vi "MC_7_12f_JW.vi"() -> ()   [LabVIEW 2011]
uses:
  <vilib>/Utility/file.llb/Read From Spreadsheet File (string).vi
  <vilib>/Utility/inputDevices.llb/keyboardAcquire.vi
  <vilib>/Utility/file.llb/Write To Spreadsheet File (DBL).vi
  <vilib>/Utility/file.llb/Write To Spreadsheet File (string).vi
  <vilib>/regexp/Match Regular Expression.xnode
panel:
  out "Rec: Temp":dbl
  out "Comments":string
  out "Folder Index":dbl caption="Length"
  out "Current \nRecord":string[](array[string])
  out "Transformer \nHeaders":string[](array[string])
  out "Current Device ID":string
  out "Column":string
  out "Row":string
  out "Rec: Concentration":dbl
  out "Rec: Solvent":string
  out "Rec: Method":string
  in  "?":T1(tab)
  out "Rec: Material":string
  in  "Treatment Concentration (mM):":dbl=30.0
  in  "Surface Treatment:":string
  in  "# Drops*:":dbl=inf
  in  "Solution Temp (C):":dbl=55.0
  in  "Relative Humidity (%):":dbl=nan
  in  "Room Temp (F):":dbl=nan
  in  "Time (s):":dbl=80.0
  out "Accel (RPM/s):":dbl
  in  "RPM:":dbl=1000.0
  in  "Wait Time (s):":dbl=10.0
  in  "Sample #:":dbl=1.0
  in  "Fabricator:":string="Jeremy"
  in  "Data File":path
  out "Data Folder":path
  in  "Image Folder":path
  out "Image File":path=path "D:/UserData/Desktop/Jeremy/WFU/Research/Programs/VI mods/Image Not Found.png"
  in  "Ramp (s):":dbl=3.0
  out "Calc: VT-Lin":dbl
  out "New: VT-Lin":dbl
  out "Rec: VT-Lin":dbl caption="VT-Lin" format="%#_3g"
  out "Calc: Trap Density-STS":dbl format="%#_4e"
  out "New: Trap Density-STS":dbl format="%#_4e"
  out "Rec: Trap Density-STS":dbl caption="Trap Density-STS" format="%#_3e"
  out "Calc: Trap Density-VT":dbl format="%#_4e"
  out "New: Trap Density-VT":dbl format="%#_4e"
  out "Rec: Trap Density-VT":dbl caption="Trap Density-VT" format="%#_3e"
  out "Calc: Onset V":dbl
  out "New: Onset":dbl
  out "Rec: Onset V":dbl caption="Onset V" format="%#_3g"
  out "Calc: Mobility-Lin":dbl format="%#_4e"
  out "New: Mobility-Lin":dbl format="%#_4e"
  out "Rec: Mobility-Lin":dbl caption="Mobility-Lin" format="%#_3e"
  out "Calc: Mobility-Sat":dbl format="%#_4e"
  out "Rec: Length":dbl caption="Length" format="%#_3g"
  out "Rec: Width":dbl caption="Width" format="%#_4g"
  out "Rec: Dielectric (d)":dbl caption="Dielectric (d)" format="%#_3g"
  out "XY Graph":cluster{dbl[], dbl[]}[](graph)
  in  "NumPts":dbl=5.0
  in  "Cancel Button":bool
  in  "Next Button":bool
  in  "Previous Button":bool
  in  "Up Button":bool
  in  "Down Button":bool
  out "Data Name:":string
  in  "Save Changes?":bool
  in  "New: Dielectric":dbl
  in  "New: Length":dbl
  in  "New: Width":dbl
  out "New: Mobility-Sat":dbl format="%#_4e"
  in  "Slide":dbl(slide) step=1.0 scale=-14.3..88.0 scale format="%#_1p"
  in  "Blank Button":bool
  in  "Zoom":i16(slide)=-3 scale=-5.0..5.0
  out "Image Out 2":T2(plugin-control)
  out "Image Out":T2(plugin-control)
  in  "Magnification":u16(ring) items=["5x", "10x", "20x", "50x", "80x"]
  out "Total Width":dbl
  out "Distances":dbl[](array[numeric])
  in  "Undo Button":bool
  in  "Remove Button":bool
  out "Rec: Mobility-Sat":dbl caption="Mobility-Sat" format="%#_3e"
  out "Index":string
  out "Image Name":string
  in  "Export":bool
  out "Calc: VT-Sat":dbl
  out "New: VT-Sat":dbl
  in  "Manual":bool
  out "XY Graph 2":cluster{dbl[], dbl[]}[](graph)
  in  "Next Button 2":bool
  in  "Previous Button 2":bool
  in  "Slide 2":dbl(slide) step=1.0 scale=-1.0..82.0 scale format="%#_1p"
  out "Calc: STS":dbl
  out "New: STS":dbl
  in  "NumPts 2":dbl=5.0 caption="NumPts"
  out "Rec: VT-Sat":dbl caption="VT-Sat" format="%#_3g"
  out "Rec: STS":dbl caption="STS" format="%#_3g"
  out "Rec: On/Off":dbl caption="On/Off" format="%#_3e"
  in  "Save Changes? 2":bool
  in  "Save Changes? 3":bool
  out "Date Recorded":string="Date Recorded" caption="Recorded"
  out "Date Created":string caption="Fabricated"
  out "String":string
  in  "No Image":path=path "D:/UserData/Desktop/Jeremy/WFU/Research/Programs/VI mods/Image Not Found.png"
  in  "Project":path=path "D:/UserData/Desktop/Jeremy/WFU/Research/Programs/Mega Awesome/DeviceData.opj"
  out "Index 2":dbl
  out "Array 8":dbl[](array[numeric])
  out "Array 7":dbl[](array[numeric])
  out "ROI Descriptor out":T3 {"Contours"."Type" items=["No Selection", "Point", "Line", "Rectangle", "Oval", "Polygon", "Freehand Region", "Annulus", "Unused2", "Unused3", "Broken Line", "Freehand Line", "Rotated Rectangle"]}
  out "ROI Descriptor":T3 {"Contours"."Type" items=["No Selection", "Point", "Line", "Rectangle", "Oval", "Polygon", "Freehand Region", "Annulus", "Unused2", "Unused3", "Broken Line", "Freehand Line", "Rotated Rectangle"]}
  out "Numeric 3":dbl
  out "Array 6":dbl[][](array[numeric])
  out "Cluster":T4
  out "Array 5":dbl[](array[numeric])
  out "Array 4":dbl[](array[numeric])
  out "Array 3":dbl[](array[numeric])
  out "Numeric 2":dbl
  out "Numeric":dbl
  out "Array 2":dbl[](array[numeric])
  out "Array":dbl[](array[numeric])
  out "MobVi Index":dbl
  in  "Row Start":dbl=20.0
  # "Data Locations"
  # "Data Location"
  # "Image Location"
  # "Sample Properties"
  # "*     Inf = Full coverage\n   NaN = Unknown or Not Applicable"
  # "Recorded"
  # "Calculated"
  # "Re-Calculated"
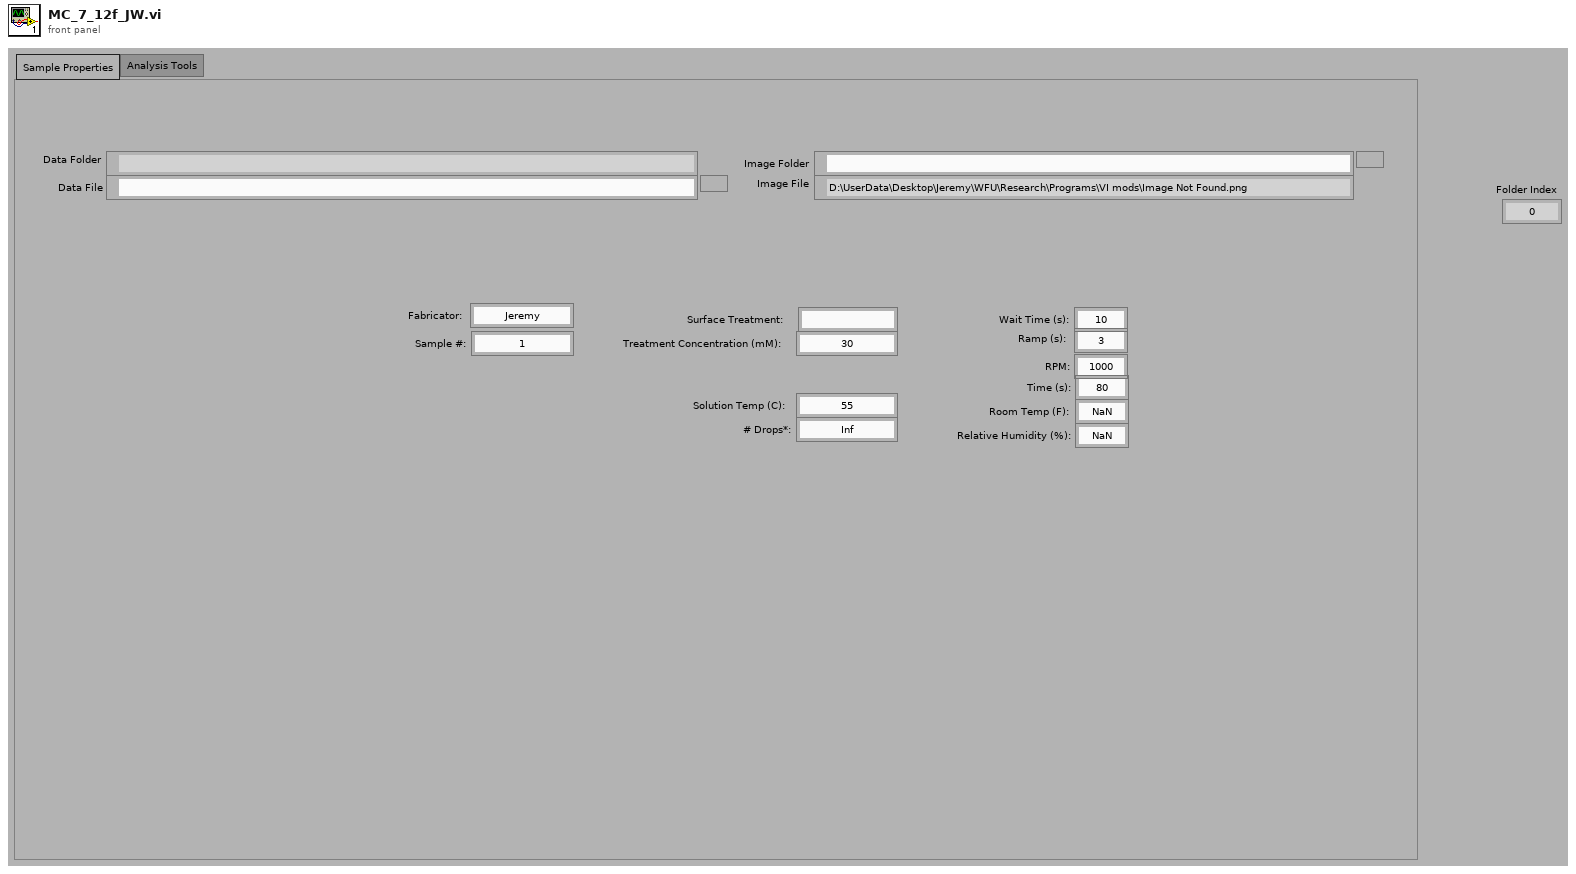
[diagram p1: front panel]
types:
  T1 = enum32{"Sample Properties", "Analysis Tools", "Current Database"}
  T2 = typedef "IMAQ Image.ctl" = refnum<image>
  T3 = typedef "ROI Descriptor" = cluster{"Global Rectangle":i32[], "Contours":cluster{"ID":enum32{"External", "Internal"}, "Type":u32, "Coordinates":i32[]}[]}
  T4 = cluster{"Numeric":dbl, "Numeric 2":dbl, "Numeric 3":dbl, "Numeric 4":dbl}
  T5 = cluster{"Mobility-Sat":dbl, "Moblitity-Lin":dbl, "On/Off":dbl, "Threshold Voltage":dbl, "Onset Voltage":dbl, "STS":dbl, "Trap Density-VT":dbl, "Trap Density-STS":dbl}
  T6 = cluster{"Date Recorded":string, "Index":string, "Length":dbl, "Width":dbl, "Sample Temp":dbl}
  T7 = cluster{"Date Created":string, "Material":string, "Solvent":string, "Concentration":dbl, "Method":string, "Dielectric (nm)":dbl, "Treatment":string, "Comments":string}
  T8 = cluster{"Mobility-Sat":dbl, "Vt-Sat":dbl, "Mobility-Lin":dbl, "Vt-Lin":dbl}
  T9 = cluster{"[0]":cluster{dbl[], dbl[]}, "[1]":cluster{dbl[], dbl[]}, "[2]":cluster{dbl[], dbl[]}, "[3]":cluster{dbl[], dbl[]}, "[4]":cluster{dbl[], dbl[]}, "[5]":cluster{dbl[], dbl[]}, "[6]":cluster{dbl[], dbl[]}, "[7]":cluster{dbl[], dbl[]}, "[8]":cluster{dbl[], dbl[]}}
  T10 = cluster{"Global Rectangle":i32[], "Contours":cluster{"Contour Type":u32, "ROI Type":u32, "Points":i32[]}[]}
  T11 = typedef "LVBoundsTypeDef.ctl" = cluster{"Width":u32, "Height":u32}
  T12 = enum16{"0", "1", "2", "3", "4", "5", "6", "7", "8", "9", "A", "B", "C", "D", "E", "F", "G", "H", "I", "J", "K", "L", "M", "N", "O", "P", "Q", "R", "S", "T", "U", "V", "W", "X", "Y", "Z", "F1", "F2", "F3", "F4", "F5", "F6", "F7", "F8", "F9", "F10", "F11", "F12", "F13", "F14", "F15", "ADD", "BACK", "BACKSLASH", "CAPITAL", "COMMA", "DECIMAL", "DELETE", "DIVIDE", "DOWN", "END", "EQUALS", "ESCAPE", "GRAVE (`)", "HOME", "INSERT", "LBRACKET", "LCONTROL", "LEFT", "L ALT", "LSHIFT", "LWIN", "MINUS", "MULTIPLY", "NEXT", "NUMLOCK", "NUMPAD_0", "NUMPAD_1", "NUMPAD_2", "NUMPAD_3", "NUMPAD_4", "NUMPAD_5", "NUMPAD_6", "NUMPAD_7", "NUMPAD_8", "NUMPAD_9", "PAUSE", "PERIOD", "PRIOR (PG UP)", "RBRACKET", "RCONTROL", "RETURN", "RIGHT", "R ALT", "RSHIFT", "RWIN", "SCROLL", "SEMICOLON", "SLASH", "SPACE", "SUBTRACT", "TAB", "UP", "ENTER (num pad)", "' (quote)"}[]
  T13 = cluster{"Contour Type":u32, "ROI Type":u32, "Points":i32[]}[]
  T14 = cluster{i32[], cluster{"Contour Type":u32, "ROI Type":u32, "Points":i32[]}[]}
  T15 = enum16{"0", "1", "2", "3", "4", "5", "6", "7", "8", "9", "A", "B", "C", "D", "E", "F", "G", "H", "I", "J", "K", "L", "M", "N", "O", "P", "Q", "R", "S", "T", "U", "V", "W", "X", "Y", "Z", "F1", "F2", "F3", "F4", "F5", "F6", "F7", "F8", "F9", "F10", "F11", "F12", "F13", "F14", "F15", "ADD", "BACK", "BACKSLASH", "CAPITAL", "COMMA", "DECIMAL", "DELETE", "DIVIDE", "DOWN", "END", "EQUALS", "ESCAPE", "GRAVE (`)", "HOME", "INSERT", "LBRACKET", "LCONTROL", "LEFT", "L ALT", "LSHIFT", "LWIN", "MINUS", "MULTIPLY", "NEXT", "NUMLOCK", "NUMPAD_0", "NUMPAD_1", "NUMPAD_2", "NUMPAD_3", "NUMPAD_4", "NUMPAD_5", "NUMPAD_6", "NUMPAD_7", "NUMPAD_8", "NUMPAD_9", "PAUSE", "PERIOD", "PRIOR (PG UP)", "RBRACKET", "RCONTROL", "RETURN", "RIGHT", "R ALT", "RSHIFT", "RWIN", "SCROLL", "SEMICOLON", "SLASH", "SPACE", "SUBTRACT", "TAB", "UP", "ENTER (num pad)", "' (quote)"}
  T16 = cluster{string, sgl, bool, bool, bool, bool, bool, bool, i32}
  T17 = cluster{i32, cluster{string, sgl, bool, bool, bool, bool, bool, bool, i32}, i32, i32}
  T18 = cluster{"Contour Type":u32, "ROI Type":u32, "Points":i32[]}
  T19 = cluster{"Points[0]":i32, "Points[1]":i32, "Points[2]":i32, "Points[3]":i32, "Points[4]":i32, "Points[5]":i32, "Points[6]":i32, "Points[7]":i32, "Points[8]":i32}
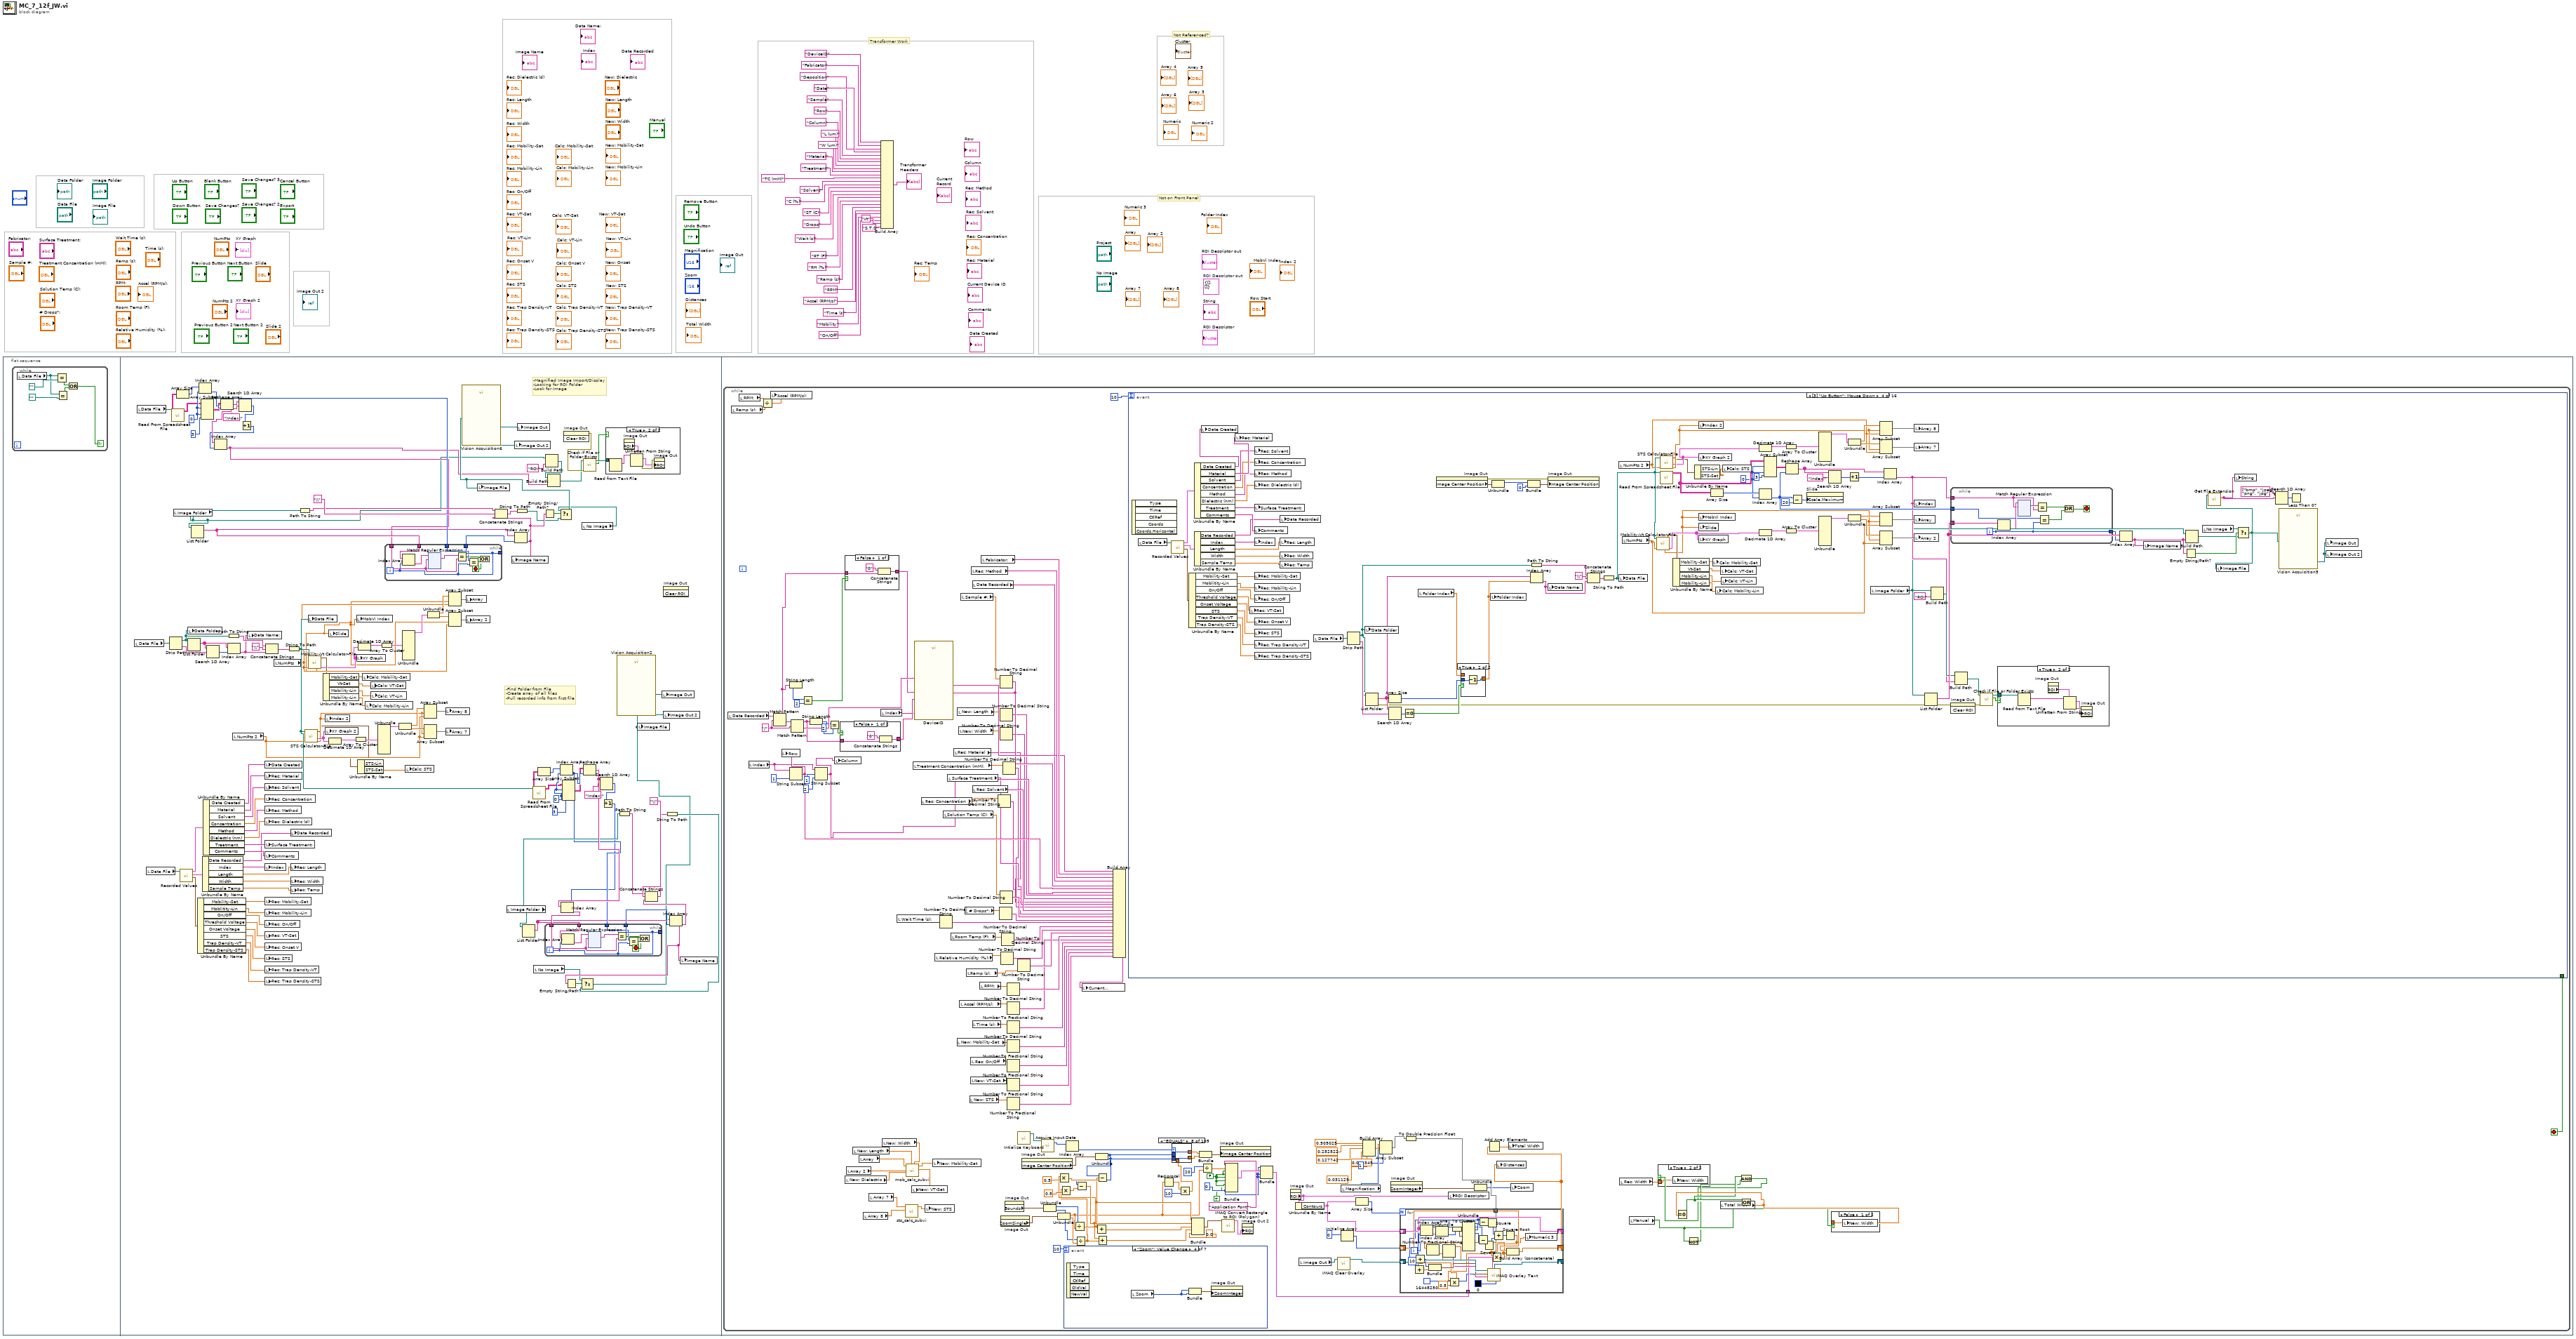
[diagram p0: block diagram]
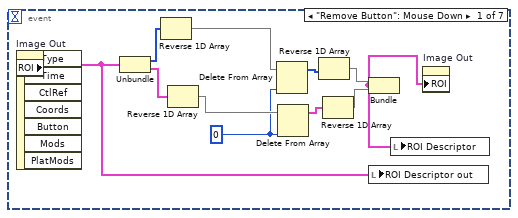
[diagram p7: hidden frame]
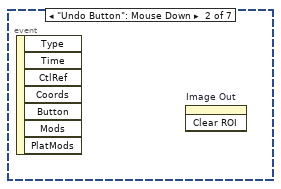
[diagram p8: hidden frame]
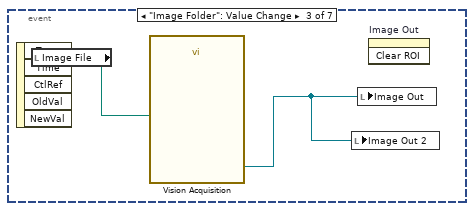
[diagram p9: hidden frame]
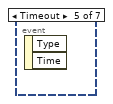
[diagram p10: hidden frame]
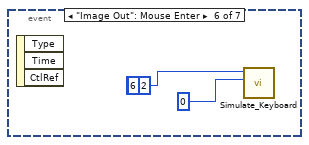
[diagram p11: hidden frame]
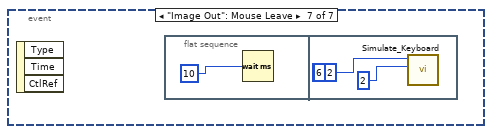
[diagram p12: hidden frame]
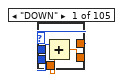
[diagram p13: hidden frame]
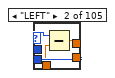
[diagram p14: hidden frame]
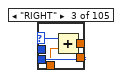
[diagram p15: hidden frame]
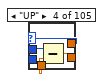
[diagram p16: hidden frame]
diagram:
  (unwired) T3 {"Global Rectangle"=[], "Contours"=[]}  # ROI Descriptor out
  # "Not Referenced?"
  # "Transformer Work"
  # "Not on Front Panel"
  n1 = flat-sequence {
    frame #0 {
      n2 = while {
        stop <- w29 continue-if-true
        n3 = local read "Data File"() -> (w31:path)
        n4 = Equal?(x=w31, y=path "") -> (x = y?=w33:bool)
        n5 = Equal?(x=w31, y=path "") -> (x = y?=w32:bool)
        n6 = Or(x=w33, y=w32) -> (x .or. y?=w29:bool)
      }
    }
    frame #1 {
      w114 = 0
      w138 = 0
      # "-Find Folder from File\n-Create array of all files\n-Pull recorded info from first file"
      # "-Magnified Image Import/Display\n-Looking for ROI Folder\n-Look for Image"
      n7 = local read "Data File"() -> (w118:path)
      n8 = local read "Data File"() -> (w133:path)
      n9 = local read "Data File"() -> (w73:path)
      n10 = Strip Path(path=w118) -> (stripped path=w119:path, name=w105:string)
      n11 = call-poly <vilib>:"Read From Spreadsheet File.vi"("file path (dialog if empty)"=w133) -> ("all rows"=w136:string[][])  [unwired: 6 in, 4 out]
      n12 = local read "Image Folder"() -> (w75:path)
      n13 = Array Size(array=w136) -> (size(s)=w137:i32[])
      n14 = call "Recorded Values.vi"("Path"=w73) -> ("Recorded Char"=w71:T5, "Recorded Prop"=w70:T6, "Fabrication Prop"=w72:T7)  [unwired: 8 in]
      n15 = local write "Data Folder"(w119) -> ()
      n16 = List Folder(path=w119) -> (filenames=w109:string[])  [unwired: 3 in, 3 out]
      n17 = List Folder(path=w75) -> (filenames=w142:string[])  [unwired: 3 in, 3 out]
      n18 = Unbundle By Name(w71) -> ("Mobility-Sat"=w57:dbl, "Moblitity-Lin"=w56:dbl, "On/Off"=w55:dbl, "Threshold Voltage"=w54:dbl, "Onset Voltage"=w53:dbl, "STS"=w52:dbl, "Trap Density-VT"=w51:dbl, "Trap Density-STS"=w50:dbl)
      n19 = Index Array(array=w137, index=w138) -> (element=w144:i32)
      n20 = Array Subset(array=w136, index (row)=w138, index (col)=w138, length (col)=3) -> (w135:string[][])  [unwired: 1 in]
      n21 = Unbundle By Name(w70) -> ("Date Recorded"=w62:string, "Index"=w61:string, "Length"=w60:dbl, "Width"=w59:dbl, "Sample Temp"=w58:dbl)
      n22 = Unbundle By Name(w72) -> ("Date Created"=w49:string, "Material"=w69:string, "Solvent"=w68:string, "Concentration"=w67:dbl, "Method"=w66:string, "Dielectric (nm)"=w65:dbl, "Treatment"=w64:string, "Comments"=w63:string)
      n23 = Search 1D Array(1D array=w109, element=w105) -> (index of element=w108:i32)  [unwired: 1 in]
      n24 = Reshape Array(w135, w144) -> (w149:string[])
      n25 = Path To String(path=w119) -> (string=w104:string)
      n26 = Index Array(array=w109, index=w108) -> (element=w74:string)
      n27 = local read "NumPts 2"() -> (w39:dbl)
      n28 = Search 1D Array(1D array=w149, element="Index:") -> (index of element=w141:i32)  [unwired: 1 in]
      n29 = Increment(x=w141) -> (x+1=w140:i32)
      n30 = Index Array(array=w149, index=w140) -> (element=w76:string)
      n31 = local write "Data Name:"(w74) -> ()
      n32 = local write "Date Created"(w49) -> ()
      n33 = local write "Rec: Material"(w69) -> ()
      n34 = local write "Rec: Solvent"(w68) -> ()
      n35 = local write "Rec: Concentration"(w67) -> ()
      n36 = local write "Rec: Method"(w66) -> ()
      n37 = local write "Rec: Dielectric (d)"(w65) -> ()
      n38 = local write "Surface Treatment:"(w64) -> ()
      n39 = local write "Comments"(w63) -> ()
      n40 = local write "Index"(w61) -> ()
      n41 = local write "Rec: Mobility-Sat"(w57) -> ()
      n42 = local write "Rec: Mobility-Lin"(w56) -> ()
      n43 = local write "Rec: On/Off"(w55) -> ()
      n44 = local write "Rec: VT-Sat"(w54) -> ()
      n45 = local write "Rec: Onset V"(w53) -> ()
      n46 = local write "Rec: STS"(w52) -> ()
      n47 = local write "Rec: Trap Density-VT"(w51) -> ()
      n48 = local write "Rec: Trap Density-STS"(w50) -> ()
      n49 = Concatenate Strings(w104, "\\", w74) -> (w106:string)
      n50 = local read "NumPts"() -> (w43:dbl)
      n51 = String To Path(string=w106) -> (path=w48:path)
      n52 = local write "Date Recorded"(w62) -> ()
      n53 = local write "Rec: Length"(w60) -> ()
      n54 = local write "Rec: Width"(w59) -> ()
      n55 = local write "Rec: Temp"(w58) -> ()
      n56 = Path To String(path=w75) -> (string=w146:string)
      n57 = call "STS Calculator-File.vi"("NumPts"=w39, "Path"=w48) -> ("STS Index-Sat"=w37:dbl, "XY Graph-Sat"=w38:cluster{dbl[], dbl[]}[], "Ouput"=w36:cluster{"STS-Sat":dbl, "STS-Lin":dbl})  [unwired: 5 in, 2 out]
      n58 = local write "Data File"(w48) -> ()
      n59 = call "Mobility-Vt Calculator-File.vi"("NumPts"=w43, "Path"=w48) -> ("XY Graph-Sat"=w41:cluster{dbl[], dbl[]}[], "Output"=w42:T8, "Index-Sat"=w40:dbl)  [unwired: 5 in, 2 out]
      n60 = Unbundle By Name(w42) -> ("Mobility-Sat"=w47:dbl, "Vt-Sat"=w46:dbl, "Mobility-Lin"=w45:dbl, "Mobility-Lin"=w44:dbl)
      n61 = local write "Index 2"(w37) -> ()
      n62 = local write "XY Graph 2"(w38) -> ()
      n63 = local write "Slide"(w40) -> ()
      n64 = Decimate 1D Array(w38) -> (w96:cluster{dbl[], dbl[]}[])  [unwired: 1 out]
      n65 = Array To Cluster(array=w96) -> (cluster=w98:T9)
      n66 = local write "MobVi Index"(w40) -> ()
      n67 = local write "XY Graph"(w41) -> ()
      n68 = Unbundle By Name(w36) -> ("STS-Sat"=w35:dbl)  [unwired: 1 out]
      n69 = Decimate 1D Array(w41) -> (w132:cluster{dbl[], dbl[]}[])  [unwired: 1 out]
      n70 = local write "Calc: Mobility-Sat"(w47) -> ()
      n71 = local write "Calc: Mobility-Lin"(w44) -> ()
      n72 = local write "Calc: VT-Sat"(w46) -> ()
      n73 = local write "Calc: VT-Lin"(w45) -> ()
      n74 = Unbundle(w98) -> ("[0]"=w97:cluster{dbl[], dbl[]})  [unwired: 8 out]
      n75 = Array To Cluster(array=w132) -> (cluster=w130:T9)
      n76 = while {
        tunnel: w142 -> [w282]
        tunnel: w76 -> [w280]
        tunnel: [w279] -> _
        tunnel: [w279] -> w143
        tunnel: w144 -> [w278]
        i -> [w279]
        stop <- w275 stop-if-true
        n77 = Index Array(array=w282, index=w279) -> (element=w283:string)
        n78 = xnode "Match Regular Expression"("input string"=w283, "regular expression"=w280) -> ("whole match"=w281:string)  [unwired: 4 in, 4 out]
        n79 = Equal?(x=w281, y=w280) -> (x = y?=w277:bool)
        n80 = Equal?(x=w278, y=w279) -> (x = y?=w276:bool)
        n81 = Or(x=w277, y=w276) -> (x .or. y?=w275:bool)
      }
      n82 = Unbundle(w97) -> (w94:dbl[], w93:dbl[])
      n83 = Unbundle(w130) -> ("[0]"=w131:cluster{dbl[], dbl[]})  [unwired: 8 out]
      n84 = local write "Calc: STS"(w35) -> ()
      n85 = Array Subset(array=w94, index=w37, length=w39) -> (w101:dbl[])
      n86 = Array Subset(array=w93, index=w37, length=w39) -> (w100:dbl[])
      n87 = Unbundle(w131) -> (w95:dbl[], w99:dbl[])
      n88 = local write "Array 8"(w101) -> ()
      n89 = local write "Array 7"(w100) -> ()
      n90 = Array Subset(array=w95, index=w40, length=w43) -> (w102:dbl[])
      n91 = Array Subset(array=w99, index=w40, length=w43) -> (w103:dbl[])
      n92 = local write "Array"(w102) -> ()
      n93 = local write "Array 2"(w103) -> ()
      n94 = local read "Image Folder"() -> (w125:path)
      n95 = Index Array(array=w142, index=w143) -> (element=w92:string)
      n96 = Concatenate Strings(w146, "\\", w92) -> (w147:string)
      n97 = local write "Image Name"(w92) -> ()
      n98 = String To Path(string=w147) -> (path=w90:path)
      n99 = List Folder(path=w125) -> (filenames=w121:string[])  [unwired: 3 in, 3 out]
      n100 = call-poly <vilib>:"Read From Spreadsheet File.vi"("file path (dialog if empty)"=w48) -> ("all rows"=w112:string[][])  [unwired: 6 in, 4 out]
      n101 = local read "No Image"() -> (w84:path)
      n102 = Array Size(array=w112) -> (size(s)=w113:i32[])
      n103 = Empty String/Path?(string/path=w92) -> (empty?=w91:bool)
      n104 = Build Path(base path=w75, name or relative path="ROI") -> (appended path=w78:path)
      n105 = Build Path(base path=w78, name or relative path=w76) -> (appended path=w77:path)
      n106 = Index Array(array=w113, index=w114) -> (element=w124:i32)
      n107 = Array Subset(array=w112, index (row)=w114, index (col)=w114, length (col)=3) -> (w111:string[][])  [unwired: 1 in]
      n108 = invoke on="Image Out" class="ImageControl" method="Clear ROI"() -> (error out=w82:errorcluster)  [unwired: 3 in, 2 out]
      n109 = local read "No Image"() -> (w83:path)
      n110 = Select(t=w83, s=w91, f=w90) -> (s? t:f=w89:path)
      n111 = call "Vision Acquisition6"("Image Path"=w89) -> ("Image Out"=w145:T2)  [unwired: 25 in, 1 out]
      n112 = local write "Image File"(w89) -> ()
      n113 = local write "Image Out 2"(w145) -> ()
      n114 = local write "Image Out"(w145) -> ()
      n115 = call <vilib>:"Check if File or Folder Exists.vi"("error in (no error)"=w82, "path"=w77) -> ("file or folder exists?"=w80:bool, "dup path"=w81:path)  [unwired: 7 in, 1 out]
      n116 = Reshape Array(w111, w124) -> (w129:string[])
      n117 = Search 1D Array(1D array=w129, element="Index:") -> (index of element=w117:i32)  [unwired: 1 in]
      n118 = Increment(x=w117) -> (x+1=w116:i32)
      n119 = Index Array(array=w129, index=w116) -> (element=w122:string)
      n120 = while {
        tunnel: w121 -> [w162]
        tunnel: w122 -> [w160]
        tunnel: [w159] -> _
        tunnel: [w159] -> w123
        tunnel: w124 -> [w158]
        i -> [w159]
        stop <- w155 stop-if-true
        n121 = Index Array(array=w162, index=w159) -> (element=w163:string)
        n122 = xnode "Match Regular Expression"("input string"=w163, "regular expression"=w160) -> ("whole match"=w161:string)  [unwired: 4 in, 4 out]
        n123 = Equal?(x=w161, y=w160) -> (x = y?=w157:bool)
        n124 = Equal?(x=w158, y=w159) -> (x = y?=w156:bool)
        n125 = Or(x=w157, y=w156) -> (x .or. y?=w155:bool)
      }
      n126 = case shown="True" w80 {
        tunnel: w81 -> [_ w150]
        frame False {
        }
        frame True {
          n127 = Read from Text File(file (use dialog)=w150) -> (text=w154:string)  [unwired: 3 in, 3 out]
          n128 = property on="Image Out" class="ImageControl"() -> ("ROI"=w151:T10)  [unwired: 2 in, 2 out]
          n129 = Unflatten From String(type=w151, binary string=w154) -> (value=w152:T10, error out=w153:errorcluster)  [unwired: 3 in, 1 out]
          n130 = property on="Image Out" class="ImageControl"(error in=w153, "ROI"=w152) -> ()  [unwired: 1 in, 2 out]
        }
      }
      n131 = Path To String(path=w125) -> (string=w126:string)
      n132 = invoke on="Image Out" class="ImageControl" method="Clear ROI"() -> ()  [unwired: 3 in, 3 out]
      n133 = Index Array(array=w121, index=w123) -> (element=w87:string)
      n134 = Empty String/Path?(string/path=w87) -> (empty?=w88:bool)
      n135 = Concatenate Strings(w126, "\\", w87) -> (w127:string)
      n136 = String To Path(string=w127) -> (path=w86:path)
      n137 = Select(t=w84, s=w88, f=w86) -> (s? t:f=w85:path)
      n138 = call "Vision Acquisition2"("Image Path"=w85) -> ("Image Out"=w120:T2)  [unwired: 25 in, 1 out]
      n139 = local write "Image File"(w85) -> ()
      n140 = local write "Image Out"(w120) -> ()
      n141 = local write "Image Out 2"(w120) -> ()
      n142 = local write "Image Name"(w87) -> ()
    }
    frame #2 {
      n143 = while {
        stop <- w542 stop-if-true
        w428 = "/"
        w492 = FALSE
        w490 = 0
        n144 = local read "Date Recorded"() -> (w431:string)
        n145 = local read "Ramp (s):"() -> (w398:dbl)
        n146 = local read "RPM:"() -> (w399:dbl)
        n147 = local read "Index"() -> (w401:string)
        n148 = Divide(x=w399, y=w398) -> (x/y=w397:dbl)
        n149 = local write "Accel (RPM/s):"(w397) -> ()
        n150 = Match Pattern(string=w431, regular expression=w428) -> (before substring=w422:string, after substring=w429:string)  [unwired: 1 in, 2 out]
        n151 = String Subset(string=w401, length (rest)=1) -> (substring=w456:string)  [unwired: 1 in]
        n152 = local write "Row"(w456) -> ()
        n153 = String Length(string=w422) -> (length=w425:i32)
        n154 = Match Pattern(string=w429, regular expression=w428) -> (before substring=w416:string, after substring=w427:string)  [unwired: 1 in, 2 out]
        n155 = Equal?(x=w425, y=2) -> (x = y?=w423:bool)
        n156 = String Length(string=w416) -> (length=w418:i32)
        n157 = String Subset(string=w401, offset (0)=1, length (rest)=2) -> (substring=w457:string)
        n158 = Equal?(x=w418, y=2) -> (x = y?=w420:bool)
        n159 = local write "Column"(w457) -> ()
        n160 = case shown="False" w420 {
          tunnel: w416 -> [w544 w546]
          tunnel: [w543 w546] -> w417
          frame False {
            n161 = Concatenate Strings("0", w544) -> (w543:string)
          }
          frame True {
          }
        }
        n162 = case shown="False" w423 {
          tunnel: w422 -> [w548 w550]
          tunnel: [w547 w550] -> w421
          frame False {
            n163 = Concatenate Strings("0", w548) -> (w547:string)
          }
          frame True {
          }
        }
        n164 = local read "New: Dielectric"() -> (w480:dbl)
        n165 = local read "Array 2"() -> (w476:dbl[])
        n166 = local read "New: Length"() -> (w478:dbl)
        n167 = local read "Array"() -> (w477:dbl[])
        n168 = local read "Array 8"() -> (w472:dbl[])
        n169 = local read "Array 7"() -> (w473:dbl[])
        n170 = local read "Index"() -> (w415:string)
        n171 = local read "New: Width"() -> (w481:dbl)
        n172 = local read "Wait Time (s):"() -> (w461:dbl)
        n173 = call "sts_calc_subvi.vi"("Array 2"=w472, "Array"=w473) -> ("STS"=w474:dbl)  [unwired: 9 in]
        n174 = call "mob_calc_subvi.vi"("Width"=w481, "Length"=w478, "Dielectric (d)"=w480, "Array 2"=w476, "Array"=w477) -> ("Vt"=w475:dbl, "Mobility"=w479:dbl)  [unwired: 4 in, 1 out]
        n175 = local write "New: VT-Sat"(w475) -> ()
        n176 = local read "Treatment Concentration (mM):"() -> (w409:dbl)
        n177 = local read "Rec: Concentration"() -> (w396:dbl)
        n178 = local write "New: STS"(w474) -> ()
        n179 = local write "New: Mobility-Sat"(w479) -> ()
        n180 = local read "Relative Humidity (%):"() -> (w406:dbl)
        n181 = Number To Decimal String(number=w461) -> (decimal integer string=w462:string)  [unwired: 1 in]
        n182 = local read "Solution Temp (C):"() -> (w450:dbl)
        n183 = local read "Surface Treatment:"() -> (w408:string)
        n184 = local read "Room Temp (F):"() -> (w454:dbl)
        n185 = local read "Rec: Material"() -> (w404:string)
        n186 = local read "New: Mobility-Sat"() -> (w443:dbl)
        n187 = local read "New: Length"() -> (w414:dbl)
        n188 = local read "New: Width"() -> (w413:dbl)
        n189 = local read "Accel (RPM/s):"() -> (w441:dbl)
        n190 = local read "Sample #:"() -> (w433:dbl)
        n191 = local read "# Drops*:"() -> (w451:dbl)
        n192 = local read "Ramp (s):"() -> (w459:dbl)
        n193 = local read "New: STS"() -> (w435:dbl)
        n194 = local read "New: VT-Sat"() -> (w437:dbl)
        n195 = local read "Rec: On/Off"() -> (w439:dbl)
        n196 = local read "Rec: Method"() -> (w434:string)
        n197 = local read "Date Recorded"() -> (w430:string)
        n198 = local read "Rec: Solvent"() -> (w410:string)
        n199 = local read "Time (s):"() -> (w446:dbl)
        n200 = local read "RPM:"() -> (w447:dbl)
        n201 = local read "Fabricator:"() -> (w455:string)
        n202 = Number To Decimal String(number=w396) -> (decimal integer string=w395:string)  [unwired: 1 in]
        n203 = Number To Decimal String(number=w451) -> (decimal integer string=w452:string)  [unwired: 1 in]
        n204 = Number To Decimal String(number=w433) -> (decimal integer string=w426:string)  [unwired: 1 in]
        n205 = call "DeviceID"("Sample"=w426, "Year"=w427, "Month"=w421, "Day"=w417, "Index"=w415) -> ("Result"=w432:string)  [unwired: 9 in, 1 out]
        n206 = Number To Decimal String(number=w414) -> (decimal integer string=w412:string)  [unwired: 1 in]
        n207 = Number To Decimal String(number=w413) -> (decimal integer string=w411:string)  [unwired: 1 in]
        n208 = Number To Decimal String(number=w450) -> (decimal integer string=w449:string)  [unwired: 1 in]
        n209 = property on="Image Out" class="ImageControl"() -> ("ZoomSingle"=w510:cluster{"X":sgl, "Y":sgl})  [unwired: 2 in, 2 out]
        n210 = Number To Decimal String(number=w406) -> (decimal integer string=w405:string)  [unwired: 1 in]
        n211 = Number To Decimal String(number=w454) -> (decimal integer string=w453:string)  [unwired: 1 in]
        n212 = Number To Decimal String(number=w409) -> (decimal integer string=w407:string)  [unwired: 1 in]
        n213 = property on="Image Out" class="ImageControl"() -> ("Bounds"=w511:T11)  [unwired: 2 in, 2 out]
        n214 = Number To Decimal String(number=w447) -> (decimal integer string=w448:string)  [unwired: 1 in]
        n215 = Number To Fractional String(number=w441) -> (F-format string=w442:string)  [unwired: 3 in]
        n216 = Number To Decimal String(number=w446) -> (decimal integer string=w445:string)  [unwired: 1 in]
        n217 = Number To Fractional String(number=w443) -> (F-format string=w444:string)  [unwired: 3 in]
        n218 = Number To Fractional String(number=w439) -> (F-format string=w440:string)  [unwired: 3 in]
        n219 = Number To Fractional String(number=w437) -> (F-format string=w438:string)  [unwired: 3 in]
        n220 = Number To Fractional String(number=w435) -> (F-format string=w436:string)  [unwired: 3 in]
        n221 = Number To Decimal String(number=w459) -> (decimal integer string=w460:string)  [unwired: 1 in]
        n222 = call <vilib>:"Intialize Keyboard.vi"() -> ("device ID"=w522:refnum<k1>)  [unwired: 10 in, 1 out]
        n223 = property on="Image Out" class="ImageControl"() -> ("Image Center Position"=w517:cluster{"X":u32, "Y":u32})  [unwired: 2 in, 2 out]
        n224 = call-poly <vilib>:"Acquire Input Data.vi"("device ID"=w522) -> ("keys pressed"=w521:T12)  [unwired: 16 in, 2 out]
        n225 = Unbundle(w511) -> ("Width"=w508:u32, "Height"=w507:u32)
        n226 = Unbundle(w510) -> ("X"=w485:sgl, "Y"=w509:sgl)
        n227 = event shown="[3] \"Zoom\": Value Change" {
          selector: _ -> [_ _ _ _ _ _ _]
          dyn-events: _ -> [_ _ _ _ _ _ _]
          timeout: 10 -> [_ _ _ _ _ _ _]
          event "Remove Button": Mouse Down {
            w555 = 0
            n228 = property on="Image Out" class="ImageControl"() -> ("ROI"=w553:T10)  [unwired: 2 in, 2 out]
            n229 = event-data() -> ()  [unwired: 1 in, 7 out]
            n230 = Unbundle(w553) -> ("Global Rectangle"=w556:i32[], "Contours"=w558:T13)
            n231 = Reverse 1D Array(array=w556) -> (reversed array=w557:i32[])
            n232 = Reverse 1D Array(array=w558) -> (reversed array=w559:T13)
            n233 = Delete From Array(array=w557, index=w555) -> (array with subset deleted=w560:i32[])  [unwired: 1 in, 1 out]
            n234 = Delete From Array(array=w559, index=w555) -> (array with subset deleted=w561:T13)  [unwired: 1 in, 1 out]
            n235 = Reverse 1D Array(array=w560) -> (reversed array=w562:i32[])
            n236 = Reverse 1D Array(array=w561) -> (reversed array=w563:T13)
            n237 = Bundle(w562, w563) -> (w554:T14)  [unwired: 1 in]
            n238 = local write "ROI Descriptor out"(w553) -> ()
            n239 = local write "ROI Descriptor"(w554) -> ()
            n240 = property on="Image Out" class="ImageControl"("ROI"=w554) -> ()  [unwired: 2 in, 2 out]
          }
          event "Undo Button": Mouse Down {
            n241 = event-data() -> ()  [unwired: 1 in, 7 out]
            n242 = invoke on="Image Out" class="ImageControl" method="Clear ROI"() -> ()  [unwired: 3 in, 3 out]
          }
          event "Image Folder": Value Change {
            n243 = event-data() -> ()  [unwired: 1 in, 5 out]
            n244 = local read "Image File"() -> (w565:path)
            n245 = call "Vision Acquisition"("Image Path"=w565) -> ("Image Out"=w564:T2)  [unwired: 25 in, 1 out]
            n246 = local write "Image Out 2"(w564) -> ()
            n247 = local write "Image Out"(w564) -> ()
            n248 = invoke on="Image Out" class="ImageControl" method="Clear ROI"() -> ()  [unwired: 3 in, 3 out]
          }
          event "Zoom": Value Change {
            n249 = event-data() -> ()  [unwired: 1 in, 5 out]
            n250 = local read "Zoom"() -> (w566:i16)
            n251 = Bundle("Zoom"=w566, "Zoom"=w566) -> (w567:cluster{"Zoom":i16, "Zoom":i16})  [unwired: 1 in]
            n252 = property on="Image Out" class="ImageControl"("ZoomInteger"=w567) -> ()  [unwired: 2 in, 2 out]
          }
          event Timeout {
            n253 = event-data() -> ()  [unwired: 1 in, 2 out]
          }
          event "Image Out": Mouse Enter {
            (unwired) 6
            n254 = event-data() -> ()  [unwired: 1 in, 3 out]
            n255 = call "Simulate_Keyboard.vi"("Action"=0, "Virtual Key"=162) -> ()  [unwired: 7 in, 1 out]
          }
          event "Image Out": Mouse Leave {
            n256 = event-data() -> ()  [unwired: 1 in, 3 out]
            n257 = flat-sequence {
              frame #0 {
                n258 = Wait (ms)(milliseconds to wait=10) -> ()  [unwired: 1 out]
              }
              frame #1 {
                (unwired) 6
                n259 = call "Simulate_Keyboard.vi"("Action"=2, "Virtual Key"=162) -> ()  [unwired: 7 in, 1 out]
              }
            }
          }
        }
        n260 = Index Array(array=w521) -> (element=w525:T15)  [unwired: 1 in]
        n261 = Divide(x=w508, y=w485) -> (x/y=w498:sgl)
        n262 = Multiply(x=w498, y=0.5) -> (x*y=w504:dbl)
        n263 = Divide(x=w507, y=w509) -> (x/y=w497:sgl)
        n264 = Multiply(x=w497, y=0.5) -> (x*y=w503:dbl)
        n265 = Unbundle(w517) -> ("X"=w499:u32, "Y"=w500:u32)
        n266 = Subtract(x=w500, y=w503) -> (x-y=w501:dbl)
        n267 = Subtract(x=w499, y=w504) -> (x-y=w502:dbl)
        n268 = Add(x=w502, y=w498) -> (x+y=w516:dbl)
        n269 = Add(x=w501, y=w497) -> (x+y=w515:dbl)
        n270 = Build Array(w432, w455, w434, w430, w426, w456, w457, w412, w411, w404, w408, w407, w410, w395, w449, w452, w462, w453, w405, w460, w448, w442, w445, w444, w440, w438, w436) -> (w458:string[])
        n271 = local write "Current \nRecord"(w458) -> ()
        n272 = event shown="[3] \"Up Button\": Mouse Down" {
          selector: _ -> [_ _ _ _ _ _ _ _ _ _ _ _ _ _ _ _]
          dyn-events: _ -> [_ _ _ _ _ _ _ _ _ _ _ _ _ _ _ _]
          timeout: 10 -> [_ _ _ _ _ _ _ _ _ _ _ _ _ _ _ _]
          tunnel: [_ _ _ _ _ _ _ _ _ _ _ _ _ TRUE _ TRUE] -> w542
          event Timeout {
            n273 = event-data() -> ()  [unwired: 1 in, 2 out]
          }
          event "Down Button": Mouse Down {
            w913 = 0
            n274 = event-data() -> ()  [unwired: 1 in, 7 out]
            n275 = local read "Data File"() -> (w863:path)
            n276 = local read "Data File"() -> (w918:path)
            n277 = call "Recorded Values.vi"("Path"=w863) -> ("Recorded Char"=w861:T5, "Recorded Prop"=w860:T6, "Fabrication Prop"=w862:T7)  [unwired: 8 in]
            n278 = Strip Path(path=w918) -> (stripped path=w909:path, name=w927:string)
            n279 = Unbundle By Name(w861) -> ("Mobility-Sat"=w847:dbl, "Moblitity-Lin"=w846:dbl, "On/Off"=w845:dbl, "Threshold Voltage"=w844:dbl, "Onset Voltage"=w843:dbl, "STS"=w842:dbl, "Trap Density-VT"=w841:dbl, "Trap Density-STS"=w840:dbl)
            n280 = local write "Data Folder"(w909) -> ()
            n281 = Unbundle By Name(w862) -> ("Date Created"=w839:string, "Material"=w859:string, "Solvent"=w858:string, "Concentration"=w857:dbl, "Method"=w856:string, "Dielectric (nm)"=w855:dbl, "Treatment"=w854:string, "Comments"=w853:string)
            n282 = Unbundle By Name(w860) -> ("Date Recorded"=w852:string, "Index"=w851:string, "Length"=w850:dbl, "Width"=w849:dbl, "Sample Temp"=w848:dbl)
            n283 = local write "Date Created"(w839) -> ()
            n284 = local write "Rec: VT-Sat"(w844) -> ()
            n285 = local write "Rec: Material"(w859) -> ()
            n286 = local write "Rec: Concentration"(w857) -> ()
            n287 = local write "Rec: Method"(w856) -> ()
            n288 = local write "Rec: Dielectric (d)"(w855) -> ()
            n289 = local write "Surface Treatment:"(w854) -> ()
            n290 = local write "Comments"(w853) -> ()
            n291 = local write "Index"(w851) -> ()
            n292 = local write "Rec: Mobility-Sat"(w847) -> ()
            n293 = local write "Rec: Mobility-Lin"(w846) -> ()
            n294 = local write "Rec: On/Off"(w845) -> ()
            n295 = local write "Rec: Onset V"(w843) -> ()
            n296 = local write "Rec: STS"(w842) -> ()
            n297 = local write "Rec: Trap Density-VT"(w841) -> ()
            n298 = local write "Rec: Trap Density-STS"(w840) -> ()
            n299 = List Folder(path=w909) -> (filenames=w923:string[], error out=w838:errorcluster)  [unwired: 3 in, 2 out]
            n300 = local write "Rec: Solvent"(w858) -> ()
            n301 = local write "Date Recorded"(w852) -> ()
            n302 = local write "Rec: Length"(w850) -> ()
            n303 = local write "Rec: Width"(w849) -> ()
            n304 = local write "Rec: Temp"(w848) -> ()
            n305 = Array Size(array=w923) -> (size(s)=w919:i32)
            n306 = Search 1D Array(1D array=w923, element=w927) -> (index of element=w920:i32)  [unwired: 1 in]
            n307 = Decrement(x=w919) -> (x-1=w921:i32)
            n308 = Equal?(x=w920, y=w921) -> (x = y?=w922:bool)
            n309 = local read "Folder Index"() -> (w865:dbl)
            n310 = case shown="False" w922 {
              tunnel: w865 -> [w1056 _]
              tunnel: [w1055 0] -> w864
              tunnel: w838 -> [w1054 w1057]
              tunnel: [w1054 w1057] -> w837
              frame False {
                n311 = Increment(x=w1056) -> (x+1=w1055:dbl)
              }
              frame True {
              }
            }
            n312 = property on="Image Out" class="ImageControl"() -> (error out=w866:errorcluster, "Image Center Position"=w870:cluster{"X":u32, "Y":u32})  [unwired: 2 in, 1 out]
            n313 = invoke on="Image Out" class="ImageControl" method="Clear ROI"() -> ()  [unwired: 3 in, 3 out]
            n314 = Unbundle(w870) -> ("X"=w868:u32)  [unwired: 1 out]
            n315 = local write "Folder Index"(w864) -> ()
            n316 = Bundle("X"=w868, 0) -> (w869:cluster{"X":u32, i32})  [unwired: 1 in]
            n317 = property on="Image Out" class="ImageControl"(error in=w866, "Image Center Position"=w869) -> ()  [unwired: 1 in, 2 out]
            n318 = Path To String(path=w909) -> (string=w928:string)
            n319 = Index Array(array=w923, index=w864) -> (element=w924:string)
            n320 = local write "Data Name:"(w924) -> ()
            n321 = Concatenate Strings(w928, "\\", w924) -> (w926:string)
            n322 = String To Path(string=w926) -> (path=w836:path)
            n323 = local read "NumPts 2"() -> (w827:dbl)
            n324 = local write "Data File"(w836) -> ()
            n325 = local read "NumPts"() -> (w831:dbl)
            n326 = call-poly <vilib>:"Read From Spreadsheet File.vi"("file path (dialog if empty)"=w836) -> ("all rows"=w915:string[][])  [unwired: 6 in, 4 out]
            n327 = call "Mobility-Vt Calculator-File.vi"("NumPts"=w831, "Path"=w836) -> ("XY Graph-Sat"=w829:cluster{dbl[], dbl[]}[], "Output"=w830:T8, "Index-Sat"=w828:dbl)  [unwired: 5 in, 2 out]
            n328 = call "STS Calculator-File.vi"("NumPts"=w827, "Path"=w836) -> ("STS Index-Sat"=w826:dbl, "XY Graph-Sat"=w825:cluster{dbl[], dbl[]}[], "Ouput"=w824:cluster{"STS-Sat":dbl, "STS-Lin":dbl})  [unwired: 5 in, 2 out]
            n329 = Unbundle By Name(w830) -> ("Mobility-Sat"=w835:dbl, "Vt-Sat"=w834:dbl, "Mobility-Lin"=w833:dbl, "Mobility-Lin"=w832:dbl)
            n330 = Unbundle By Name(w824) -> ("STS-Sat"=w823:dbl)  [unwired: 1 out]
            n331 = local write "Index 2"(w826) -> ()
            n332 = local write "XY Graph 2"(w825) -> ()
            n333 = local write "MobVi Index"(w828) -> ()
            n334 = local write "Slide"(w828) -> ()
            n335 = local write "XY Graph"(w829) -> ()
            n336 = Array Size(array=w915) -> (size(s)=w914:i32[])
            n337 = local write "Calc: Mobility-Sat"(w835) -> ()
            n338 = local write "Calc: STS"(w823) -> ()
            n339 = local write "Calc: Mobility-Lin"(w832) -> ()
            n340 = local write "Calc: VT-Sat"(w834) -> ()
            n341 = local write "Calc: VT-Lin"(w833) -> ()
            n342 = Index Array(array=w914, index=w913) -> (element=w895:i32)
            n343 = Decimate 1D Array(w825) -> (w889:cluster{dbl[], dbl[]}[])  [unwired: 1 out]
            n344 = Decimate 1D Array(w829) -> (w899:cluster{dbl[], dbl[]}[])  [unwired: 1 out]
            n345 = Array Subset(array=w915, index (row)=w913, index (col)=w913, length (col)=3) -> (w916:string[][])  [unwired: 1 in]
            n346 = Array To Cluster(array=w889) -> (cluster=w887:T9)
            n347 = Array To Cluster(array=w899) -> (cluster=w901:T9)
            n348 = Reshape Array(w916, w895) -> (w902:string[])
            n349 = Subtract(x=w895, y=20) -> (x-y=w894:i32)
            n350 = property on="Slide" class="Slide (strict)"("Scale.Maximum"=w894) -> ()  [unwired: 2 in, 2 out]
            n351 = Unbundle(w887) -> ("[0]"=w888:cluster{dbl[], dbl[]})  [unwired: 8 out]
            n352 = Unbundle(w901) -> ("[0]"=w900:cluster{dbl[], dbl[]})  [unwired: 8 out]
            n353 = Search 1D Array(1D array=w902, element="Index:") -> (index of element=w910:i32)  [unwired: 1 in]
            n354 = local read "Image Folder"() -> (w872:path)
            n355 = Increment(x=w910) -> (x+1=w911:i32)
            n356 = Unbundle(w888) -> (w886:dbl[], w885:dbl[])
            n357 = Unbundle(w900) -> (w891:dbl[], w890:dbl[])
            n358 = Array Subset(array=w886, index=w826, length=w827) -> (w893:dbl[])
            n359 = Array Subset(array=w885, index=w826, length=w827) -> (w892:dbl[])
            n360 = Array Subset(array=w891, index=w828, length=w831) -> (w898:dbl[])
            n361 = Array Subset(array=w890, index=w828, length=w831) -> (w897:dbl[])
            n362 = Index Array(array=w902, index=w911) -> (element=w874:string)
            n363 = List Folder(path=w872, error in=w837) -> (filenames=w908:string[], error out=w875:errorcluster)  [unwired: 2 in, 2 out]
            n364 = Build Path(base path=w872, name or relative path="ROI") -> (appended path=w871:path)
            n365 = while {
              tunnel: w908 -> [w941]
              tunnel: w874 -> [w939]
              tunnel: [w938] -> _
              tunnel: [w938] -> w907
              tunnel: w895 -> [w937]
              i -> [w938]
              stop <- w934 stop-if-true
              n366 = Index Array(array=w941, index=w938) -> (element=w942:string)
              n367 = xnode "Match Regular Expression"("input string"=w942, "regular expression"=w939) -> ("whole match"=w940:string)  [unwired: 4 in, 4 out]
              n368 = Equal?(x=w940, y=w939) -> (x = y?=w936:bool)
              n369 = Equal?(x=w937, y=w938) -> (x = y?=w935:bool)
              n370 = Or(x=w936, y=w935) -> (x .or. y?=w934:bool)
            }
            n371 = local write "Array 8"(w893) -> ()
            n372 = local write "Array 7"(w892) -> ()
            n373 = local write "Array"(w898) -> ()
            n374 = local write "Array 2"(w897) -> ()
            n375 = invoke on="Image Out" class="ImageControl" method="Clear ROI"(error in=w875) -> (error out=w878:errorcluster)  [unwired: 2 in, 2 out]
            n376 = Build Path(base path=w871, name or relative path=w874) -> (appended path=w879:path)
            n377 = call <vilib>:"Check if File or Folder Exists.vi"("error in (no error)"=w878, "path"=w879) -> ("file or folder exists?"=w876:bool, "dup path"=w877:path)  [unwired: 7 in, 1 out]
            n378 = case shown="True" w876 {
              tunnel: w877 -> [_ w929]
              frame False {
              }
              frame True {
                n379 = Read from Text File(file (use dialog)=w929) -> (text=w933:string)  [unwired: 3 in, 3 out]
                n380 = property on="Image Out" class="ImageControl"() -> ("ROI"=w930:T10)  [unwired: 2 in, 2 out]
                n381 = Unflatten From String(type=w930, binary string=w933) -> (value=w931:T10, error out=w932:errorcluster)  [unwired: 3 in, 1 out]
                n382 = property on="Image Out" class="ImageControl"(error in=w932, "ROI"=w931) -> ()  [unwired: 1 in, 2 out]
              }
            }
            n383 = Path To String(path=w872) -> (string=w905:string)
            n384 = Index Array(array=w908, index=w907) -> (element=w883:string)
            n385 = local write "Image Name"(w883) -> ()
            n386 = Concatenate Strings(w905, "\\", w883) -> (w904:string)
            n387 = String To Path(string=w904) -> (path=w882:path)
            n388 = Empty String/Path?(string/path=w883) -> (empty?=w884:bool)
            n389 = local read "No Image"() -> (w880:path)
            n390 = Select(t=w880, s=w884, f=w882) -> (s? t:f=w881:path)
            n391 = local write "Image File"(w881) -> ()
            n392 = call "Vision Acquisition4"("Image Path"=w881) -> ("Image Out"=w906:T2)  [unwired: 25 in, 1 out]
            n393 = local write "Image Out"(w906) -> ()
            n394 = local write "Image Out 2"(w906) -> ()
          }
          event "Data File": Value Change {
            w1149 = 0
            n395 = event-data() -> ()  [unwired: 1 in, 5 out]
            n396 = local read "Data File"() -> (w1098:path)
            n397 = call "Recorded Values.vi"("Path"=w1098) -> ("Recorded Char"=w1096:T5, "Recorded Prop"=w1095:T6, "Fabrication Prop"=w1097:T7)  [unwired: 8 in]
            n398 = Unbundle By Name(w1096) -> ("Mobility-Sat"=w1082:dbl, "Moblitity-Lin"=w1081:dbl, "On/Off"=w1080:dbl, "Threshold Voltage"=w1079:dbl, "Onset Voltage"=w1078:dbl, "STS"=w1077:dbl, "Trap Density-VT"=w1076:dbl, "Trap Density-STS"=w1075:dbl)
            n399 = Unbundle By Name(w1097) -> ("Date Created"=w1074:string, "Material"=w1094:string, "Solvent"=w1093:string, "Concentration"=w1092:dbl, "Method"=w1091:string, "Dielectric (nm)"=w1090:dbl, "Treatment"=w1089:string, "Comments"=w1088:string)
            n400 = Unbundle By Name(w1095) -> ("Date Recorded"=w1087:string, "Index"=w1086:string, "Length"=w1085:dbl, "Width"=w1084:dbl, "Sample Temp"=w1083:dbl)
            n401 = local write "Date Created"(w1074) -> ()
            n402 = local read "Data File"() -> (w1145:path)
            n403 = local write "Rec: Material"(w1094) -> ()
            n404 = local write "Rec: VT-Sat"(w1079) -> ()
            n405 = local write "Rec: Concentration"(w1092) -> ()
            n406 = local write "Rec: Method"(w1091) -> ()
            n407 = local write "Rec: Dielectric (d)"(w1090) -> ()
            n408 = local write "Surface Treatment:"(w1089) -> ()
            n409 = local write "Comments"(w1088) -> ()
            n410 = local write "Index"(w1086) -> ()
            n411 = local write "Rec: Mobility-Sat"(w1082) -> ()
            n412 = local write "Rec: Mobility-Lin"(w1081) -> ()
            n413 = local write "Rec: On/Off"(w1080) -> ()
            n414 = local write "Rec: Onset V"(w1078) -> ()
            n415 = local write "Rec: STS"(w1077) -> ()
            n416 = local write "Rec: Trap Density-VT"(w1076) -> ()
            n417 = local write "Rec: Trap Density-STS"(w1075) -> ()
            n418 = Strip Path(path=w1145) -> (stripped path=w1144:path, name=w1158:string)
            n419 = local write "Rec: Solvent"(w1093) -> ()
            n420 = local write "Date Recorded"(w1087) -> ()
            n421 = local write "Rec: Length"(w1085) -> ()
            n422 = local write "Rec: Width"(w1084) -> ()
            n423 = local write "Rec: Temp"(w1083) -> ()
            n424 = local write "Data Folder"(w1144) -> ()
            n425 = property on="Image Out" class="ImageControl"() -> (error out=w1100:errorcluster, "Image Center Position"=w1104:cluster{"X":u32, "Y":u32})  [unwired: 2 in, 1 out]
            n426 = List Folder(path=w1144) -> (filenames=w1154:string[], error out=w1110:errorcluster)  [unwired: 3 in, 2 out]
            n427 = Search 1D Array(1D array=w1154, element=w1158) -> (index of element=w1099:i32)  [unwired: 1 in]
            n428 = local write "Folder Index"(w1099) -> ()
            n429 = Unbundle(w1104) -> ("X"=w1102:u32)  [unwired: 1 out]
            n430 = Path To String(path=w1144) -> (string=w1159:string)
            n431 = Index Array(array=w1154, index=w1099) -> (element=w1155:string)
            n432 = Bundle("X"=w1102, 0) -> (w1103:cluster{"X":u32, i32})  [unwired: 1 in]
            n433 = local write "Data Name:"(w1155) -> ()
            n434 = property on="Image Out" class="ImageControl"(error in=w1100, "Image Center Position"=w1103) -> ()  [unwired: 1 in, 2 out]
            n435 = Concatenate Strings(w1159, "\\", w1155) -> (w1157:string)
            n436 = String To Path(string=w1157) -> (path=w1073:path)
            n437 = local read "NumPts 2"() -> (w1063:dbl)
            n438 = local write "Data File"(w1073) -> ()
            n439 = local read "NumPts"() -> (w1064:dbl)
            n440 = call-poly <vilib>:"Read From Spreadsheet File.vi"("file path (dialog if empty)"=w1073) -> ("all rows"=w1151:string[][])  [unwired: 6 in, 4 out]
            n441 = call "STS Calculator-File.vi"("NumPts"=w1063, "Path"=w1073) -> ("STS Index-Sat"=w1061:dbl, "XY Graph-Sat"=w1062:cluster{dbl[], dbl[]}[], "Ouput"=w1060:cluster{"STS-Sat":dbl, "STS-Lin":dbl})  [unwired: 5 in, 2 out]
            n442 = call "Mobility-Vt Calculator-File.vi"("NumPts"=w1064, "Path"=w1073) -> ("XY Graph-Sat"=w1067:cluster{dbl[], dbl[]}[], "Output"=w1065:T8, "Index-Sat"=w1066:dbl)  [unwired: 5 in, 2 out]
            n443 = Unbundle By Name(w1065) -> ("Mobility-Sat"=w1072:dbl, "Vt-Sat"=w1071:dbl, "Mobility-Lin"=w1070:dbl, "Mobility-Lin"=w1069:dbl)
            n444 = local write "Index 2"(w1061) -> ()
            n445 = local write "XY Graph 2"(w1062) -> ()
            n446 = Unbundle By Name(w1060) -> ("STS-Sat"=w1059:dbl)  [unwired: 1 out]
            n447 = local write "MobVi Index"(w1066) -> ()
            n448 = Array Size(array=w1151) -> (size(s)=w1150:i32[])
            n449 = local write "Slide"(w1066) -> ()
            n450 = local write "Calc: Mobility-Sat"(w1072) -> ()
            n451 = local write "Calc: Mobility-Lin"(w1069) -> ()
            n452 = local write "Calc: VT-Sat"(w1071) -> ()
            n453 = local write "Calc: VT-Lin"(w1070) -> ()
            n454 = local write "Calc: STS"(w1059) -> ()
            n455 = Decimate 1D Array(w1062) -> (w1125:cluster{dbl[], dbl[]}[])  [unwired: 1 out]
            n456 = Index Array(array=w1150, index=w1149) -> (element=w1131:i32)
            n457 = Decimate 1D Array(w1067) -> (w1134:cluster{dbl[], dbl[]}[])  [unwired: 1 out]
            n458 = local write "XY Graph"(w1067) -> ()
            n459 = Array Subset(array=w1151, index (row)=w1149, index (col)=w1149, length (col)=3) -> (w1152:string[][])  [unwired: 1 in]
            n460 = Array To Cluster(array=w1125) -> (cluster=w1123:T9)
            n461 = Array To Cluster(array=w1134) -> (cluster=w1136:T9)
            n462 = Reshape Array(w1152, w1131) -> (w1137:string[])
            n463 = Subtract(x=w1131, y=20) -> (x-y=w1129:i32)
            n464 = property on="Slide" class="Slide (strict)"("Scale.Maximum"=w1129) -> ()  [unwired: 2 in, 2 out]
            n465 = Unbundle(w1123) -> ("[0]"=w1124:cluster{dbl[], dbl[]})  [unwired: 8 out]
            n466 = Unbundle(w1136) -> ("[0]"=w1135:cluster{dbl[], dbl[]})  [unwired: 8 out]
            n467 = Search 1D Array(1D array=w1137, element="Index:") -> (index of element=w1146:i32)  [unwired: 1 in]
            n468 = local read "NumPts"() -> (w1068:dbl)
            n469 = Increment(x=w1146) -> (x+1=w1147:i32)
            n470 = Unbundle(w1124) -> (w1121:dbl[], w1120:dbl[])
            n471 = Unbundle(w1135) -> (w1122:dbl[], w1126:dbl[])
            n472 = local read "Image Folder"() -> (w1106:path)
            n473 = Array Subset(array=w1121, index=w1061, length=w1063) -> (w1128:dbl[])
            n474 = Array Subset(array=w1120, index=w1061, length=w1063) -> (w1127:dbl[])
            n475 = Array Subset(array=w1122, index=w1066, length=w1068) -> (w1133:dbl[])
            n476 = Array Subset(array=w1126, index=w1066, length=w1068) -> (w1132:dbl[])
            n477 = Index Array(array=w1137, index=w1147) -> (element=w1108:string)
            n478 = local write "Array 8"(w1128) -> ()
            n479 = local write "Array 7"(w1127) -> ()
            n480 = local write "Index"(w1108) -> ()
            n481 = local write "Array"(w1133) -> ()
            n482 = local write "Array 2"(w1132) -> ()
            n483 = List Folder(path=w1106, error in=w1110) -> (filenames=w1142:string[], error out=w1109:errorcluster)  [unwired: 2 in, 2 out]
            n484 = Build Path(base path=w1106, name or relative path="ROI") -> (appended path=w1105:path)
            n485 = while {
              tunnel: w1142 -> [w1172]
              tunnel: w1108 -> [w1170]
              tunnel: [w1169] -> _
              tunnel: [w1169] -> w1141
              tunnel: w1131 -> [w1168]
              i -> [w1169]
              stop <- w1165 stop-if-true
              n486 = Index Array(array=w1172, index=w1169) -> (element=w1173:string)
              n487 = xnode "Match Regular Expression"("input string"=w1173, "regular expression"=w1170) -> ("whole match"=w1171:string)  [unwired: 4 in, 4 out]
              n488 = Equal?(x=w1171, y=w1170) -> (x = y?=w1167:bool)
              n489 = Equal?(x=w1168, y=w1169) -> (x = y?=w1166:bool)
              n490 = Or(x=w1167, y=w1166) -> (x .or. y?=w1165:bool)
            }
            n491 = invoke on="Image Out" class="ImageControl" method="Clear ROI"(error in=w1109) -> (error out=w1113:errorcluster)  [unwired: 2 in, 2 out]
            n492 = Build Path(base path=w1105, name or relative path=w1108) -> (appended path=w1114:path)
            n493 = call <vilib>:"Check if File or Folder Exists.vi"("error in (no error)"=w1113, "path"=w1114) -> ("file or folder exists?"=w1111:bool, "dup path"=w1112:path)  [unwired: 7 in, 1 out]
            n494 = case shown="True" w1111 {
              tunnel: w1112 -> [_ w1160]
              frame False {
              }
              frame True {
                n495 = Read from Text File(file (use dialog)=w1160) -> (text=w1164:string)  [unwired: 3 in, 3 out]
                n496 = property on="Image Out" class="ImageControl"() -> ("ROI"=w1161:T10)  [unwired: 2 in, 2 out]
                n497 = Unflatten From String(type=w1161, binary string=w1164) -> (value=w1162:T10, error out=w1163:errorcluster)  [unwired: 3 in, 1 out]
                n498 = property on="Image Out" class="ImageControl"(error in=w1163, "ROI"=w1162) -> ()  [unwired: 1 in, 2 out]
              }
            }
            n499 = invoke on="Image Out" class="ImageControl" method="Clear ROI"() -> ()  [unwired: 3 in, 3 out]
            n500 = Path To String(path=w1106) -> (string=w1140:string)
            n501 = Index Array(array=w1142, index=w1141) -> (element=w1118:string)
            n502 = Concatenate Strings(w1140, "\\", w1118) -> (w1139:string)
            n503 = local write "Image Name"(w1118) -> ()
            n504 = String To Path(string=w1139) -> (path=w1117:path)
            n505 = Empty String/Path?(string/path=w1118) -> (empty?=w1119:bool)
            n506 = local read "No Image"() -> (w1115:path)
            n507 = Select(t=w1115, s=w1119, f=w1117) -> (s? t:f=w1116:path)
            n508 = local write "Image File"(w1116) -> ()
            n509 = call "Vision Acquisition3"("Image Path"=w1116) -> ("Image Out"=w1143:T2)  [unwired: 25 in, 1 out]
            n510 = local write "Image Out"(w1143) -> ()
            n511 = local write "Image Out 2"(w1143) -> ()
          }
          event "Up Button": Mouse Down {
            w1376 = 0
            n512 = event-data() -> ()  [unwired: 1 in, 5 out]
            n513 = local read "Data File"() -> (w1323:path)
            n514 = call "Recorded Values.vi"("Path"=w1323) -> ("Recorded Char"=w1321:T5, "Recorded Prop"=w1320:T6, "Fabrication Prop"=w1322:T7)  [unwired: 8 in]
            n515 = Unbundle By Name(w1321) -> ("Mobility-Sat"=w1307:dbl, "Moblitity-Lin"=w1306:dbl, "On/Off"=w1305:dbl, "Threshold Voltage"=w1304:dbl, "Onset Voltage"=w1303:dbl, "STS"=w1302:dbl, "Trap Density-VT"=w1301:dbl, "Trap Density-STS"=w1300:dbl)
            n516 = Unbundle By Name(w1322) -> ("Date Created"=w1299:string, "Material"=w1319:string, "Solvent"=w1318:string, "Concentration"=w1317:dbl, "Method"=w1316:string, "Dielectric (nm)"=w1315:dbl, "Treatment"=w1314:string, "Comments"=w1313:string)
            n517 = Unbundle By Name(w1320) -> ("Date Recorded"=w1312:string, "Index"=w1311:string, "Length"=w1310:dbl, "Width"=w1309:dbl, "Sample Temp"=w1308:dbl)
            n518 = local write "Date Created"(w1299) -> ()
            n519 = local write "Rec: Material"(w1319) -> ()
            n520 = local write "Rec: VT-Sat"(w1304) -> ()
            n521 = local write "Rec: Solvent"(w1318) -> ()
            n522 = local write "Rec: Concentration"(w1317) -> ()
            n523 = local write "Rec: Method"(w1316) -> ()
            n524 = local write "Rec: Dielectric (d)"(w1315) -> ()
            n525 = local write "Surface Treatment:"(w1314) -> ()
            n526 = local write "Comments"(w1313) -> ()
            n527 = local write "Index"(w1311) -> ()
            n528 = local write "Rec: Mobility-Sat"(w1307) -> ()
            n529 = local write "Rec: Mobility-Lin"(w1306) -> ()
            n530 = local write "Rec: On/Off"(w1305) -> ()
            n531 = local write "Rec: Onset V"(w1303) -> ()
            n532 = local write "Rec: STS"(w1302) -> ()
            n533 = local write "Rec: Trap Density-VT"(w1301) -> ()
            n534 = local write "Rec: Trap Density-STS"(w1300) -> ()
            n535 = local write "Date Recorded"(w1312) -> ()
            n536 = local write "Rec: Length"(w1310) -> ()
            n537 = local write "Rec: Width"(w1309) -> ()
            n538 = local write "Rec: Temp"(w1308) -> ()
            n539 = local read "Data File"() -> (w1372:path)
            n540 = Strip Path(path=w1372) -> (stripped path=w1371:path, name=w1387:string)
            n541 = local write "Data Folder"(w1371) -> ()
            n542 = List Folder(path=w1371) -> (filenames=w1381:string[], error out=w1338:errorcluster)  [unwired: 3 in, 2 out]
            n543 = Array Size(array=w1381) -> (size(s)=w1326:i32)
            n544 = Search 1D Array(1D array=w1381, element=w1387) -> (index of element=w1382:i32)  [unwired: 1 in]
            n545 = Equal To 0?(x=w1382) -> (x = 0?=w1383:bool)
            n546 = local read "Folder Index"() -> (w1325:dbl)
            n547 = property on="Image Out" class="ImageControl"() -> (error out=w1328:errorcluster, "Image Center Position"=w1332:cluster{"X":u32, "Y":u32})  [unwired: 2 in, 1 out]
            n548 = case shown="True" w1383 {
              tunnel: w1325 -> [w1515 _]
              tunnel: [w1514 w1516] -> w1324
              tunnel: w1326 -> [_ w1517]
              frame False {
                n549 = Decrement(x=w1515) -> (x-1=w1514:dbl)
              }
              frame True {
                n550 = Decrement(x=w1517) -> (x-1=w1516:i32)
              }
            }
            n551 = local write "Folder Index"(w1324) -> ()
            n552 = Unbundle(w1332) -> ("X"=w1330:u32)  [unwired: 1 out]
            n553 = Bundle("X"=w1330, 0) -> (w1331:cluster{"X":u32, i32})  [unwired: 1 in]
            n554 = Path To String(path=w1371) -> (string=w1388:string)
            n555 = Index Array(array=w1381, index=w1324) -> (element=w1384:string)
            n556 = local write "Data Name:"(w1384) -> ()
            n557 = property on="Image Out" class="ImageControl"(error in=w1328, "Image Center Position"=w1331) -> ()  [unwired: 1 in, 2 out]
            n558 = Concatenate Strings(w1388, "\\", w1384) -> (w1386:string)
            n559 = String To Path(string=w1386) -> (path=w1298:path)
            n560 = local read "NumPts 2"() -> (w1289:dbl)
            n561 = local write "Data File"(w1298) -> ()
            n562 = local read "NumPts"() -> (w1293:dbl)
            n563 = call "Mobility-Vt Calculator-File.vi"("NumPts"=w1293, "Path"=w1298) -> ("XY Graph-Sat"=w1291:cluster{dbl[], dbl[]}[], "Output"=w1292:T8, "Index-Sat"=w1290:dbl)  [unwired: 5 in, 2 out]
            n564 = call "STS Calculator-File.vi"("NumPts"=w1289, "Path"=w1298) -> ("STS Index-Sat"=w1288:dbl, "XY Graph-Sat"=w1287:cluster{dbl[], dbl[]}[], "Ouput"=w1286:cluster{"STS-Sat":dbl, "STS-Lin":dbl})  [unwired: 5 in, 2 out]
            n565 = call-poly <vilib>:"Read From Spreadsheet File.vi"("file path (dialog if empty)"=w1298) -> ("all rows"=w1378:string[][])  [unwired: 6 in, 4 out]
            n566 = Unbundle By Name(w1292) -> ("Mobility-Sat"=w1297:dbl, "Vt-Sat"=w1296:dbl, "Mobility-Lin"=w1295:dbl, "Mobility-Lin"=w1294:dbl)
            n567 = Unbundle By Name(w1286) -> ("STS-Sat"=w1285:dbl)  [unwired: 1 out]
            n568 = local write "Index 2"(w1288) -> ()
            n569 = local write "XY Graph 2"(w1287) -> ()
            n570 = local write "MobVi Index"(w1290) -> ()
            n571 = local write "Slide"(w1290) -> ()
            n572 = local write "XY Graph"(w1291) -> ()
            n573 = Array Size(array=w1378) -> (size(s)=w1377:i32[])
            n574 = local write "Calc: Mobility-Sat"(w1297) -> ()
            n575 = local write "Calc: Mobility-Lin"(w1294) -> ()
            n576 = local write "Calc: VT-Sat"(w1296) -> ()
            n577 = local write "Calc: VT-Lin"(w1295) -> ()
            n578 = local write "Calc: STS"(w1285) -> ()
            n579 = Decimate 1D Array(w1287) -> (w1355:cluster{dbl[], dbl[]}[])  [unwired: 1 out]
            n580 = Index Array(array=w1377, index=w1376) -> (element=w1361:i32)
            n581 = Decimate 1D Array(w1291) -> (w1365:cluster{dbl[], dbl[]}[])  [unwired: 1 out]
            n582 = Array Subset(array=w1378, index (row)=w1376, index (col)=w1376, length (col)=3) -> (w1379:string[][])  [unwired: 1 in]
            n583 = Array To Cluster(array=w1355) -> (cluster=w1353:T9)
            n584 = Array To Cluster(array=w1365) -> (cluster=w1367:T9)
            n585 = Reshape Array(w1379, w1361) -> (w1368:string[])
            n586 = Subtract(x=w1361, y=20) -> (x-y=w1360:i32)
            n587 = property on="Slide" class="Slide (strict)"("Scale.Maximum"=w1360) -> ()  [unwired: 2 in, 2 out]
            n588 = Unbundle(w1353) -> ("[0]"=w1354:cluster{dbl[], dbl[]})  [unwired: 8 out]
            n589 = Unbundle(w1367) -> ("[0]"=w1366:cluster{dbl[], dbl[]})  [unwired: 8 out]
            n590 = Search 1D Array(1D array=w1368, element="Index:") -> (index of element=w1373:i32)  [unwired: 1 in]
            n591 = Increment(x=w1373) -> (x+1=w1374:i32)
            n592 = Unbundle(w1354) -> (w1352:dbl[], w1351:dbl[])
            n593 = Unbundle(w1366) -> (w1359:dbl[], w1358:dbl[])
            n594 = local read "Image Folder"() -> (w1327:path)
            n595 = Array Subset(array=w1352, index=w1288, length=w1289) -> (w1357:dbl[])
            n596 = Array Subset(array=w1351, index=w1288, length=w1289) -> (w1356:dbl[])
            n597 = Array Subset(array=w1359, index=w1290, length=w1293) -> (w1364:dbl[])
            n598 = Array Subset(array=w1358, index=w1290, length=w1293) -> (w1363:dbl[])
            n599 = Index Array(array=w1368, index=w1374) -> (element=w1334:string)
            n600 = local write "Array 8"(w1357) -> ()
            n601 = local write "Array 7"(w1356) -> ()
            n602 = local write "Index"(w1334) -> ()
            n603 = local write "Array"(w1364) -> ()
            n604 = local write "Array 2"(w1363) -> ()
            n605 = List Folder(path=w1327, error in=w1338) -> (filenames=w1370:string[], error out=w1337:errorcluster)  [unwired: 2 in, 2 out]
            n606 = Build Path(base path=w1327, name or relative path="ROI") -> (appended path=w1335:path)
            n607 = while {
              tunnel: w1370 -> [w1401]
              tunnel: w1334 -> [w1399]
              tunnel: [w1398] -> w1369
              tunnel: w1361 -> [w1397]
              i -> [w1398]
              stop <- w1394 stop-if-true
              n608 = Index Array(array=w1401, index=w1398) -> (element=w1402:string)
              n609 = xnode "Match Regular Expression"("input string"=w1402, "regular expression"=w1399) -> ("whole match"=w1400:string)  [unwired: 4 in, 4 out]
              n610 = Equal?(x=w1400, y=w1399) -> (x = y?=w1396:bool)
              n611 = Equal?(x=w1397, y=w1398) -> (x = y?=w1395:bool)
              n612 = Or(x=w1396, y=w1395) -> (x .or. y?=w1394:bool)
            }
            n613 = invoke on="Image Out" class="ImageControl" method="Clear ROI"(error in=w1337) -> (error out=w1341:errorcluster)  [unwired: 2 in, 2 out]
            n614 = Build Path(base path=w1335, name or relative path=w1334) -> (appended path=w1333:path)
            n615 = call <vilib>:"Check if File or Folder Exists.vi"("error in (no error)"=w1341, "path"=w1333) -> ("file or folder exists?"=w1339:bool, "dup path"=w1340:path)  [unwired: 7 in, 1 out]
            n616 = case shown="True" w1339 {
              tunnel: w1340 -> [_ w1389]
              frame False {
              }
              frame True {
                n617 = Read from Text File(file (use dialog)=w1389) -> (text=w1393:string)  [unwired: 3 in, 3 out]
                n618 = property on="Image Out" class="ImageControl"() -> ("ROI"=w1390:T10)  [unwired: 2 in, 2 out]
                n619 = Unflatten From String(type=w1390, binary string=w1393) -> (value=w1391:T10, error out=w1392:errorcluster)  [unwired: 3 in, 1 out]
                n620 = property on="Image Out" class="ImageControl"(error in=w1392, "ROI"=w1391) -> ()  [unwired: 1 in, 2 out]
              }
            }
            n621 = Index Array(array=w1370, index=w1369) -> (element=w1343:string)
            n622 = local write "Image Name"(w1343) -> ()
            n623 = Empty String/Path?(string/path=w1343) -> (empty?=w1350:bool)
            n624 = Build Path(base path=w1327, name or relative path=w1343) -> (appended path=w1342:path)
            n625 = local read "No Image"() -> (w1349:path)
            n626 = Select(t=w1349, s=w1350, f=w1342) -> (s? t:f=w1344:path)
            n627 = call <vilib>:"Get File Extension.vi"("file"=w1344) -> ("lowercase file extension"=w1346:string)  [unwired: 7 in, 3 out]
            n628 = local write "Image File"(w1344) -> ()
            n629 = local write "String"(w1346) -> ()
            n630 = Search 1D Array(1D array=string[] ["bmp", "jpeg", "png", "jpg", "gif"], element=w1346) -> (index of element=w1345:i32)  [unwired: 1 in]
            n631 = call "Vision Acquisition5"("Image Path"=w1344) -> ("Image Out"=w1348:T2)  [unwired: 25 in, 1 out]
            n632 = Less Than 0?(x=w1345) -> ()  [unwired: 1 out]
            n633 = local write "Image Out"(w1348) -> ()
            n634 = local write "Image Out 2"(w1348) -> ()
          }
          event "Save Changes? 3": Mouse Down {
            n635 = event-data() -> ()  [unwired: 1 in, 7 out]
            n636 = local read "Image Folder"() -> (w1518:path)
            n637 = Build Path(base path=w1518, name or relative path="ROI") -> (appended path=w1525:path)
            n638 = call <vilib>:"Check if File or Folder Exists.vi"("path"=w1525) -> ("file or folder exists?"=w1527:bool, "dup path"=w1524:path)  [unwired: 8 in, 1 out]
            n639 = case shown="False" w1527 {
              tunnel: w1524 -> [w1529 w1530]
              tunnel: [w1528 w1530] -> w1519
              frame False {
                n640 = Create Folder(path (use dialog)=w1529) -> (created path=w1528:path)  [unwired: 2 in, 2 out]
              }
              frame True {
              }
            }
            n641 = local read "Index"() -> (w1521:string)
            n642 = property on="Image Out" class="ImageControl"() -> ("ROI"=w1523:T10)  [unwired: 2 in, 2 out]
            n643 = Build Path(base path=w1519, name or relative path=w1521) -> (appended path=w1520:path)
            n644 = Flatten To String(anything=w1523) -> (data string=w1522:string)  [unwired: 3 in, 2 out]
            n645 = Write to Text File(file (use dialog)=w1520, text=w1522) -> ()  [unwired: 2 in, 3 out]
          }
          event "Next Button": Mouse Down {
            n646 = event-data() -> ()  [unwired: 1 in, 5 out]
            n647 = local read "XY Graph"() -> (w1543:cluster{dbl[], dbl[]}[])
            n648 = Decimate 1D Array(w1543) -> (w1539:cluster{dbl[], dbl[]}[], w1538:cluster{dbl[], dbl[]}[])
            n649 = Array To Cluster(array=w1539) -> (cluster=w1549:T9)
            n650 = local read "MobVi Index"() -> (w1545:dbl)
            n651 = Unbundle(w1549) -> ("[0]"=w1548:cluster{dbl[], dbl[]})  [unwired: 8 out]
            n652 = local read "NumPts"() -> (w1544:dbl)
            n653 = Unbundle(w1548) -> (w1547:dbl[], w1546:dbl[])
            n654 = Increment(x=w1545) -> (x+1=w1540:dbl)
            n655 = local read "New: Dielectric"() -> (w1534:dbl)
            n656 = local read "New: Length"() -> (w1533:dbl)
            n657 = local read "New: Width"() -> (w1532:dbl)
            n658 = local write "MobVi Index"(w1540) -> ()
            n659 = Array Subset(array=w1547, index=w1540, length=w1544) -> (w1536:dbl[])
            n660 = Array Subset(array=w1546, index=w1540, length=w1544) -> (w1535:dbl[])
            n661 = local write "Array"(w1536) -> ()
            n662 = local write "Array 2"(w1535) -> ()
            n663 = call "mob_calc_subvi.vi"("Width"=w1532, "Length"=w1533, "Dielectric (d)"=w1534, "Array 2"=w1535, "Array"=w1536) -> ("Vt"=w1531:dbl, "Mobility"=w1537:dbl)  [unwired: 4 in, 1 out]
            n664 = Bundle(w1536, w1535) -> (w1542:cluster{dbl[], dbl[]})  [unwired: 1 in]
            n665 = local write "New: VT-Sat"(w1531) -> ()
            n666 = local write "New: Mobility-Sat"(w1537) -> ()
            n667 = Build Array (concatenate)(w1539, w1538, w1542) -> (w1541:cluster{dbl[], dbl[]}[])
            n668 = local write "XY Graph"(w1541) -> ()
          }
          event "Next Button 2": Mouse Down {
            n669 = event-data() -> ()  [unwired: 1 in, 7 out]
            n670 = local read "XY Graph 2"() -> (w1558:cluster{dbl[], dbl[]}[])
            n671 = Decimate 1D Array(w1558) -> (w1554:cluster{dbl[], dbl[]}[], w1553:cluster{dbl[], dbl[]}[])
            n672 = Array To Cluster(array=w1554) -> (cluster=w1564:T9)
            n673 = local read "Index 2"() -> (w1560:dbl)
            n674 = Unbundle(w1564) -> ("[0]"=w1563:cluster{dbl[], dbl[]})  [unwired: 8 out]
            n675 = local read "NumPts 2"() -> (w1559:dbl)
            n676 = Unbundle(w1563) -> (w1562:dbl[], w1561:dbl[])
            n677 = Increment(x=w1560) -> (x+1=w1555:dbl)
            n678 = local write "Index 2"(w1555) -> ()
            n679 = Array Subset(array=w1562, index=w1555, length=w1559) -> (w1551:dbl[])
            n680 = Array Subset(array=w1561, index=w1555, length=w1559) -> (w1550:dbl[])
            n681 = local write "Array 8"(w1551) -> ()
            n682 = Bundle(w1551, w1550) -> (w1557:cluster{dbl[], dbl[]})  [unwired: 1 in]
            n683 = call "sts_calc_subvi.vi"("Array 2"=w1551, "Array"=w1550) -> ("STS"=w1552:dbl)  [unwired: 9 in]
            n684 = local write "Array 7"(w1550) -> ()
            n685 = Build Array (concatenate)(w1554, w1553, w1557) -> (w1556:cluster{dbl[], dbl[]}[])
            n686 = local write "New: STS"(w1552) -> ()
            n687 = local write "XY Graph 2"(w1556) -> ()
          }
          event "Previous Button 2": Mouse Down {
            n688 = event-data() -> ()  [unwired: 1 in, 7 out]
            n689 = local read "XY Graph 2"() -> (w1574:cluster{dbl[], dbl[]}[])
            n690 = Decimate 1D Array(w1574) -> (w1571:cluster{dbl[], dbl[]}[], w1570:cluster{dbl[], dbl[]}[])
            n691 = Array To Cluster(array=w1571) -> (cluster=w1579:T9)
            n692 = local read "Index 2"() -> (w1567:dbl)
            n693 = Unbundle(w1579) -> ("[0]"=w1578:cluster{dbl[], dbl[]})  [unwired: 8 out]
            n694 = local read "NumPts 2"() -> (w1575:dbl)
            n695 = Unbundle(w1578) -> (w1577:dbl[], w1576:dbl[])
            n696 = Decrement(x=w1567) -> (x-1=w1568:dbl)
            n697 = local write "Index 2"(w1568) -> ()
            n698 = Array Subset(array=w1577, index=w1568, length=w1575) -> (w1565:dbl[])
            n699 = Array Subset(array=w1576, index=w1568, length=w1575) -> (w1566:dbl[])
            n700 = local write "Array 8"(w1565) -> ()
            n701 = Bundle(w1565, w1566) -> (w1573:cluster{dbl[], dbl[]})  [unwired: 1 in]
            n702 = call "sts_calc_subvi.vi"("Array 2"=w1565, "Array"=w1566) -> ("STS"=w1569:dbl)  [unwired: 9 in]
            n703 = local write "Array 7"(w1566) -> ()
            n704 = Build Array (concatenate)(w1571, w1570, w1573) -> (w1572:cluster{dbl[], dbl[]}[])
            n705 = local write "New: STS"(w1569) -> ()
            n706 = local write "XY Graph 2"(w1572) -> ()
          }
          event "Previous Button": Mouse Down {
            n707 = event-data() -> ()  [unwired: 1 in, 5 out]
            n708 = local read "XY Graph"() -> (w1593:cluster{dbl[], dbl[]}[])
            n709 = Decimate 1D Array(w1593) -> (w1590:cluster{dbl[], dbl[]}[], w1589:cluster{dbl[], dbl[]}[])
            n710 = Array To Cluster(array=w1590) -> (cluster=w1598:T9)
            n711 = local read "MobVi Index"() -> (w1588:dbl)
            n712 = Unbundle(w1598) -> ("[0]"=w1597:cluster{dbl[], dbl[]})  [unwired: 8 out]
            n713 = local read "NumPts"() -> (w1594:dbl)
            n714 = Unbundle(w1597) -> (w1596:dbl[], w1595:dbl[])
            n715 = Decrement(x=w1588) -> (x-1=w1587:dbl)
            n716 = local read "New: Dielectric"() -> (w1581:dbl)
            n717 = local read "New: Length"() -> (w1582:dbl)
            n718 = local read "New: Width"() -> (w1583:dbl)
            n719 = local write "MobVi Index"(w1587) -> ()
            n720 = Array Subset(array=w1596, index=w1587, length=w1594) -> (w1586:dbl[])
            n721 = Array Subset(array=w1595, index=w1587, length=w1594) -> (w1585:dbl[])
            n722 = local write "Array"(w1586) -> ()
            n723 = local write "Array 2"(w1585) -> ()
            n724 = call "mob_calc_subvi.vi"("Width"=w1583, "Length"=w1582, "Dielectric (d)"=w1581, "Array 2"=w1585, "Array"=w1586) -> ("Vt"=w1580:dbl, "Mobility"=w1584:dbl)  [unwired: 4 in, 1 out]
            n725 = Bundle(w1586, w1585) -> (w1592:cluster{dbl[], dbl[]})  [unwired: 1 in]
            n726 = local write "New: VT-Sat"(w1580) -> ()
            n727 = Build Array (concatenate)(w1590, w1589, w1592) -> (w1591:cluster{dbl[], dbl[]}[])
            n728 = local write "New: Mobility-Sat"(w1584) -> ()
            n729 = local write "XY Graph"(w1591) -> ()
          }
          event "Slide": Value Change {
            n730 = event-data() -> ()  [unwired: 1 in, 5 out]
            n731 = local read "XY Graph"() -> (w1611:cluster{dbl[], dbl[]}[])
            n732 = Decimate 1D Array(w1611) -> (w1608:cluster{dbl[], dbl[]}[], w1607:cluster{dbl[], dbl[]}[])
            n733 = Array To Cluster(array=w1608) -> (cluster=w1616:T9)
            n734 = Unbundle(w1616) -> ("[0]"=w1615:cluster{dbl[], dbl[]})  [unwired: 8 out]
            n735 = local read "NumPts"() -> (w1612:dbl)
            n736 = local read "Slide"() -> (w1600:dbl)
            n737 = Unbundle(w1615) -> (w1614:dbl[], w1613:dbl[])
            n738 = local read "New: Dielectric"() -> (w1601:dbl)
            n739 = local read "New: Length"() -> (w1602:dbl)
            n740 = local read "New: Width"() -> (w1603:dbl)
            n741 = local write "MobVi Index"(w1600) -> ()
            n742 = Array Subset(array=w1614, index=w1600, length=w1612) -> (w1606:dbl[])
            n743 = Array Subset(array=w1613, index=w1600, length=w1612) -> (w1605:dbl[])
            n744 = local write "Array"(w1606) -> ()
            n745 = local write "Array 2"(w1605) -> ()
            n746 = call "mob_calc_subvi.vi"("Width"=w1603, "Length"=w1602, "Dielectric (d)"=w1601, "Array 2"=w1605, "Array"=w1606) -> ("Vt"=w1599:dbl, "Mobility"=w1604:dbl)  [unwired: 4 in, 1 out]
            n747 = Bundle(w1606, w1605) -> (w1610:cluster{dbl[], dbl[]})  [unwired: 1 in]
            n748 = local write "New: VT-Sat"(w1599) -> ()
            n749 = Build Array (concatenate)(w1608, w1607, w1610) -> (w1609:cluster{dbl[], dbl[]}[])
            n750 = local write "New: Mobility-Sat"(w1604) -> ()
            n751 = local write "XY Graph"(w1609) -> ()
          }
          event "Slide 2": Value Change {
            n752 = event-data() -> ()  [unwired: 1 in, 5 out]
            n753 = local read "XY Graph 2"() -> (w1625:cluster{dbl[], dbl[]}[])
            n754 = Decimate 1D Array(w1625) -> (w1622:cluster{dbl[], dbl[]}[], w1621:cluster{dbl[], dbl[]}[])
            n755 = Array To Cluster(array=w1622) -> (cluster=w1630:T9)
            n756 = Unbundle(w1630) -> ("[0]"=w1629:cluster{dbl[], dbl[]})  [unwired: 8 out]
            n757 = local read "NumPts 2"() -> (w1626:dbl)
            n758 = local read "Slide 2"() -> (w1620:dbl)
            n759 = Unbundle(w1629) -> (w1628:dbl[], w1627:dbl[])
            n760 = local write "Index 2"(w1620) -> ()
            n761 = Array Subset(array=w1628, index=w1620, length=w1626) -> (w1618:dbl[])
            n762 = Array Subset(array=w1627, index=w1620, length=w1626) -> (w1617:dbl[])
            n763 = local write "Array 8"(w1618) -> ()
            n764 = call "sts_calc_subvi.vi"("Array 2"=w1618, "Array"=w1617) -> ("STS"=w1619:dbl)  [unwired: 9 in]
            n765 = Bundle(w1618, w1617) -> (w1624:cluster{dbl[], dbl[]})  [unwired: 1 in]
            n766 = local write "Array 7"(w1617) -> ()
            n767 = local write "New: STS"(w1619) -> ()
            n768 = Build Array (concatenate)(w1622, w1621, w1624) -> (w1623:cluster{dbl[], dbl[]}[])
            n769 = local write "XY Graph 2"(w1623) -> ()
          }
          event "Save Changes?": Mouse Down {
            n770 = event-data() -> ()  [unwired: 1 in, 5 out]
            n771 = flat-sequence {
              tunnel: [w1661] -> w1636
              tunnel: [w1660] -> w1634
              tunnel: [w1660] -> w1633
              tunnel: [w1643] -> w1631
              tunnel: w1636 -> [w1775]
              tunnel: [w1776] -> w1635
              tunnel: w1634 -> [w1776]
              tunnel: w1633 -> [w1774]
              tunnel: [w1772] -> w1632
              tunnel: w1631 -> [w1772]
              tunnel: w1635 -> [w1781]
              tunnel: w1632 -> [w1780]
              frame #0 {
                w1648 = -1
                w1641 = "S.T.S. (V/decade):"
                w1642 = "Threshold V (V):"
                (unwired) 3
                w1646 = 1
                n772 = local read "Rec: Temp"() -> (w1639:dbl)
                n773 = Equal To 0?(x=w1639) -> (x = 0?=w1638:bool)
                n774 = case shown="False" w1638 {
                  tunnel: [w1687 ""] -> w1637
                  frame False {
                    n775 = local read "Rec: Temp"() -> (w1689:dbl)
                    n776 = Number To Decimal String(number=w1689) -> (decimal integer string=w1686:string)  [unwired: 1 in]
                    n777 = Concatenate Strings("_", w1686, "K") -> (w1687:string)
                  }
                  frame True {
                  }
                }
                n778 = flat-sequence {
                  tunnel: [w1703] -> w1640
                  tunnel: w1640 -> [w1720]
                  frame #0 {
                    # "Makes Empty File for Transformer Data"
                    n779 = local read "Data Folder"() -> (w1692:path)
                    n780 = Build Path(base path=w1692, name or relative path="Stats") -> (appended path=w1694:path)
                    n781 = call <vilib>:"Check if File or Folder Exists.vi"("path"=w1694) -> ("file or folder exists?"=w1695:bool, "dup path"=w1696:path)  [unwired: 8 in, 1 out]
                    n782 = case shown="False" w1695 {
                      tunnel: [w1700 w1702] -> w1697
                      tunnel: w1696 -> [w1701 w1702]
                      frame False {
                        n783 = Create Folder(path (use dialog)=w1701) -> (created path=w1700:path)  [unwired: 2 in, 2 out]
                      }
                      frame True {
                      }
                    }
                    n784 = Build Path(base path=w1697, name or relative path="Tranformer Data.txt") -> (appended path=w1699:path)
                    n785 = call-poly <vilib>:"Write To Spreadsheet File.vi"("append to file? (new file:F)"=TRUE, "file path (dialog if empty)"=w1699) -> ()  [unwired: 6 in, 1 out]
                  }
                  frame #1 {
                    # "Adds Headers if they don't exist"
                    n786 = Concatenate Strings("Stats\\", "Tranformer Data.txt") -> (w1710:string)
                    n787 = local read "Data Folder"() -> (w1709:path)
                    n788 = Build Path(base path=w1709, name or relative path=w1710) -> (appended path=w1703:path)
                    n789 = call-poly <vilib>:"Read From Spreadsheet File.vi"("file path (dialog if empty)"=w1703) -> ("first row"=w1708:string[])  [unwired: 6 in, 4 out]
                    n790 = Search 1D Array(1D array=w1708, element="DeviceID") -> (index of element=w1706:i32)  [unwired: 1 in]
                    n791 = Equal?(x=w1706, y=0) -> (x = y?=w1704:bool)
                    n792 = case shown="False" w1704 {
                      tunnel: w1703 -> [w1714 _]
                      frame False {
                        n793 = local read "Transformer \nHeaders"() -> (w1713:string[])
                        n794 = call-poly <vilib>:"Write To Spreadsheet File.vi"("1D data"=w1713, "file path (dialog if empty)"=w1714) -> ()  [unwired: 6 in, 1 out]
                      }
                      frame True {
                      }
                    }
                  }
                  frame #2 {
                    # "Adds current device if it doesn't exist"
                    n795 = local read "Current \nRecord"() -> (w1719:string[])
                    n796 = Index Array(array=w1719, index=0) -> (element=w1718:string)
                    n797 = Concatenate Strings("Stats\\", "Tranformer Data.txt") -> (w1723:string)
                    n798 = local read "Data Folder"() -> (w1722:path)
                    n799 = local write "Current Device ID"(w1718) -> ()
                    n800 = local read "Current Device ID"() -> (w1728:string)
                    n801 = Build Path(base path=w1722, name or relative path=w1723) -> (appended path=w1721:path)
                    n802 = call-poly <vilib>:"Read From Spreadsheet File.vi"("file path (dialog if empty)"=w1721) -> ("all rows"=w1715:string[][])  [unwired: 6 in, 4 out]
                    n803 = Index Array(array=w1715, index (col)=0) -> (element=w1716:string[])  [unwired: 1 in]
                    n804 = Search 1D Array(1D array=w1716, element=w1728) -> (index of element=w1717:i32)  [unwired: 1 in]
                    n805 = Equal?(x=w1717, y=-1) -> (x = y?=w1730:bool)
                    n806 = case shown="False" w1730 {
                      tunnel: w1720 -> [w1733 w1744]
                      tunnel: w1717 -> [w1736 _]
                      tunnel: w1715 -> [w1737 _]
                      frame False {
                        n807 = local read "Current \nRecord"() -> (w1735:string[])
                        n808 = Replace Array Subset(array=w1737, new element=w1735, index (row)=w1736) -> (w1734:string[][])  [unwired: 1 in]
                        n809 = flat-sequence {
                          tunnel: w1733 -> [w1738]
                          tunnel: w1734 -> [w1739]
                          tunnel: [w1739] -> w1732
                          tunnel: [w1738] -> w1731
                          tunnel: w1732 -> [w1741]
                          tunnel: w1731 -> [w1740]
                          frame #0 {
                            n810 = Delete(path (use dialog)=w1738) -> ()  [unwired: 4 in, 3 out]
                          }
                          frame #1 {
                            n811 = call-poly <vilib>:"Write To Spreadsheet File.vi"("append to file? (new file:F)"=TRUE, "2D data"=w1741, "file path (dialog if empty)"=w1740) -> ()  [unwired: 5 in, 1 out]
                          }
                        }
                      }
                      frame True {
                        n812 = local read "Current \nRecord"() -> (w1743:string[])
                        n813 = call-poly <vilib>:"Write To Spreadsheet File.vi"("append to file? (new file:F)"=TRUE, "1D data"=w1743, "file path (dialog if empty)"=w1744) -> ()  [unwired: 5 in, 1 out]
                      }
                    }
                  }
                }
                n814 = local read "New: Length"() -> (w1672:dbl)
                n815 = local read "Data File"() -> (w1661:path)
                n816 = call-poly <vilib>:"Read From Spreadsheet File.vi"("file path (dialog if empty)"=w1661) -> ("all rows"=w1653:string[][])  [unwired: 6 in, 4 out]
                n817 = Number To Fractional String(number=w1672) -> (F-format string=w1664:string)  [unwired: 3 in]
                n818 = local read "New: Width"() -> (w1674:dbl)
                n819 = Array Size(array=w1653) -> (size(s)=w1655:i32[])
                n820 = local read "New: Mobility-Sat"() -> (w1683:dbl)
                n821 = Replace Array Subset(array=w1653, new element=w1664, index (row)=12, index (col)=w1646) -> (w1668:string[][])
                n822 = Number To Decimal String(number=w1672) -> (decimal integer string=w1671:string)  [unwired: 1 in]
                n823 = Number To Fractional String(number=w1674) -> (F-format string=w1675:string)  [unwired: 3 in]
                n824 = Number To Decimal String(number=w1674) -> (decimal integer string=w1673:string)  [unwired: 1 in]
                n825 = Array Subset(array=w1653, index (row)=0, index (col)=0) -> (w1659:string[][])  [unwired: 2 in]
                n826 = Index Array(array=w1655, index=0) -> (element=w1654:i32)
                n827 = local read "Index"() -> (w1677:string)
                n828 = Reshape Array(w1659, w1654) -> (w1647:string[])
                n829 = Strip Path(path=w1661) -> (stripped path=w1682:path)  [unwired: 1 out]
                n830 = call "Build Text"("Temp"=w1637, "Index"=w1677, "Length"=w1671, "Width"=w1673) -> ("Result"=w1678:string)  [unwired: 10 in, 1 out]
                n831 = Search 1D Array(1D array=w1647, element=w1641) -> (index of element=w1652:i32)  [unwired: 1 in]
                n832 = Search 1D Array(1D array=w1647, element=w1642) -> (index of element=w1651:i32)  [unwired: 1 in]
                n833 = Replace Array Subset(array=w1668, new element=w1675, index (row)=13, index (col)=w1646) -> (w1670:string[][])
                n834 = Path To String(path=w1682) -> (string=w1680:string)
                n835 = local read "New: Dielectric"() -> (w1684:dbl)
                n836 = Number To Fractional String(number=w1683) -> (F-format string=w1662:string)  [unwired: 3 in]
                n837 = Equal?(x=w1652, y=w1648) -> (x = y?=w1650:bool)
                n838 = Equal?(x=w1651, y=w1648) -> (x = y?=w1649:bool)
                n839 = Replace Array Subset(array=w1670, new element=w1662, index (row)=15, index (col)=w1646) -> (w1669:string[][])
                n840 = Number To Fractional String(number=w1684) -> (F-format string=w1663:string)  [unwired: 3 in]
                n841 = Concatenate Strings(w1680, "\\", w1678) -> (w1679:string)
                n842 = String To Path(string=w1679) -> (path=w1660:path)
                n843 = Replace Array Subset(array=w1669, new element=w1663, index (row)=7, index (col)=w1646) -> (w1645:string[][])
                n844 = case shown="True" w1649 {
                  tunnel: w1651 -> [_ _]
                  tunnel: w1645 -> [w1762 w1770]
                  tunnel: [w1761 w1769] -> w1644
                  tunnel: w1642 -> [_ w1768]
                  frame False {
                    n845 = local read "New: VT-Sat"() -> (w1764:dbl)
                    n846 = Number To Fractional String(number=w1764) -> (F-format string=w1760:string)  [unwired: 3 in]
                    n847 = Replace Array Subset(array=w1762, new element=w1760, index (row)=17, index (col)=1) -> (w1761:string[][])
                  }
                  frame True {
                    n848 = local read "New: VT-Sat"() -> (w1771:dbl)
                    n849 = Number To Fractional String(number=w1771) -> (F-format string=w1767:string)  [unwired: 3 in]
                    n850 = Build Array(w1768, w1767) -> (w1766:string[])
                    n851 = Insert Into Array(array=w1770, index (row)=17, new element=w1766) -> (w1769:string[][])  [unwired: 1 in]
                  }
                }
                n852 = case shown="True" w1650 {
                  tunnel: w1652 -> [_ _]
                  tunnel: w1644 -> [w1749 w1757]
                  tunnel: [w1748 w1756] -> w1643
                  tunnel: w1641 -> [_ w1754]
                  frame False {
                    n853 = local read "New: STS"() -> (w1751:dbl)
                    n854 = Number To Fractional String(number=w1751) -> (F-format string=w1747:string)  [unwired: 3 in]
                    n855 = Replace Array Subset(array=w1749, new element=w1747, index (row)=18, index (col)=1) -> (w1748:string[][])
                  }
                  frame True {
                    n856 = local read "New: STS"() -> (w1758:dbl)
                    n857 = Number To Fractional String(number=w1758) -> (F-format string=w1755:string)  [unwired: 3 in]
                    n858 = Build Array(w1754, w1755) -> (w1753:string[])
                    n859 = Insert Into Array(array=w1757, index (row)=18, new element=w1753) -> (w1756:string[][])  [unwired: 1 in]
                  }
                }
              }
              frame #1 {
                n860 = Equal?(x=w1775, y=w1774) -> (x = y?=w1773:bool)
                n861 = case shown="False" w1773 {
                  tunnel: w1775 -> [w1779 _]
                  tunnel: w1774 -> [w1778 _]
                  frame False {
                    n862 = Move(source path=w1779, 9:TRUE, 10:w1778) -> ()  [unwired: 2 in, 3 out]
                  }
                  frame True {
                  }
                }
              }
              frame #2 {
                n863 = local write "Data File"(w1781) -> ()
                n864 = call-poly <vilib>:"Write To Spreadsheet File.vi"("2D data"=w1780, "file path (dialog if empty)"=w1781) -> ()  [unwired: 6 in, 1 out]
              }
            }
          }
          event "Save Changes? 2": Mouse Down {
            n865 = event-data() -> ()  [unwired: 1 in, 5 out]
            n866 = local read "Data File"() -> (w1806:path)
            n867 = call "Recorded Values.vi"("Path"=w1806) -> ("Recorded Char"=w1804:T5, "Recorded Prop"=w1803:T6, "Fabrication Prop"=w1805:T7)  [unwired: 8 in]
            n868 = Unbundle By Name(w1804) -> ("Mobility-Sat"=w1790:dbl, "Moblitity-Lin"=w1789:dbl, "On/Off"=w1788:dbl, "Threshold Voltage"=w1787:dbl, "Onset Voltage"=w1786:dbl, "STS"=w1785:dbl, "Trap Density-VT"=w1784:dbl, "Trap Density-STS"=w1783:dbl)
            n869 = Unbundle By Name(w1803) -> ("Date Recorded"=w1795:string, "Index"=w1794:string, "Length"=w1793:dbl, "Width"=w1792:dbl, "Sample Temp"=w1791:dbl)
            n870 = Unbundle By Name(w1805) -> ("Date Created"=w1782:string, "Material"=w1802:string, "Solvent"=w1801:string, "Concentration"=w1800:dbl, "Method"=w1799:string, "Dielectric (nm)"=w1798:dbl, "Treatment"=w1797:string, "Comments"=w1796:string)
            n871 = local write "Rec: VT-Sat"(w1787) -> ()
            n872 = local write "Date Created"(w1782) -> ()
            n873 = local write "Rec: Material"(w1802) -> ()
            n874 = local write "Rec: Solvent"(w1801) -> ()
            n875 = local write "Rec: Concentration"(w1800) -> ()
            n876 = local write "Rec: Method"(w1799) -> ()
            n877 = local write "Rec: Dielectric (d)"(w1798) -> ()
            n878 = local write "Surface Treatment:"(w1797) -> ()
            n879 = local write "Comments"(w1796) -> ()
            n880 = local write "Index"(w1794) -> ()
            n881 = local write "Rec: Mobility-Sat"(w1790) -> ()
            n882 = local write "Rec: Mobility-Lin"(w1789) -> ()
            n883 = local write "Rec: On/Off"(w1788) -> ()
            n884 = local write "Rec: Onset V"(w1786) -> ()
            n885 = local write "Rec: STS"(w1785) -> ()
            n886 = local write "Rec: Trap Density-VT"(w1784) -> ()
            n887 = local write "Rec: Trap Density-STS"(w1783) -> ()
            n888 = local write "Date Recorded"(w1795) -> ()
            n889 = local write "Rec: Length"(w1793) -> ()
            n890 = local write "Rec: Width"(w1792) -> ()
            n891 = local write "Rec: Temp"(w1791) -> ()
            n892 = stacked-sequence {
              seq-local: [w1886 _ _ _ _] -> [_ w1945 _ _ _]
              seq-local: [w1885 _ _ _ _] -> [_ w1946 _ _ _]
              seq-local: [w1885 _ _ _ _] -> [_ w1944 _ _ _]
              seq-local: [w1868 _ _ _ _] -> [_ w1942 _ _ _]
              seq-local: [_ w1946 _ _ _] -> [_ _ w1951 _ _]
              seq-local: [_ w1942 _ _ _] -> [_ _ w1950 _ _]
              frame #0 {
                w1873 = -1
                w1866 = "STS (V/decade):"
                w1867 = "Threshold V (V):"
                (unwired) 3
                w1871 = 1
                n893 = local read "Rec: Temp"() -> (w1865:dbl)
                n894 = local read "New: Length"() -> (w1897:dbl)
                n895 = local read "Data File"() -> (w1886:path)
                n896 = Equal To 0?(x=w1865) -> (x = 0?=w1864:bool)
                n897 = case shown="False" w1864 {
                  tunnel: [w1911 ""] -> w1863
                  frame False {
                    n898 = local read "Rec: Temp"() -> (w1914:dbl)
                    n899 = Number To Decimal String(number=w1914) -> (decimal integer string=w1913:string)  [unwired: 1 in]
                    n900 = Concatenate Strings("_", w1913, "K") -> (w1911:string)
                  }
                  frame True {
                  }
                }
                n901 = call-poly <vilib>:"Read From Spreadsheet File.vi"("file path (dialog if empty)"=w1886) -> ("all rows"=w1878:string[][])  [unwired: 6 in, 4 out]
                n902 = Number To Fractional String(number=w1897) -> (F-format string=w1889:string)  [unwired: 3 in]
                n903 = local read "New: Width"() -> (w1899:dbl)
                n904 = local read "New: Mobility-Sat"() -> (w1908:dbl)
                n905 = Replace Array Subset(array=w1878, new element=w1889, index (row)=12, index (col)=w1871) -> (w1893:string[][])
                n906 = Number To Fractional String(number=w1899) -> (F-format string=w1900:string)  [unwired: 3 in]
                n907 = Number To Decimal String(number=w1897) -> (decimal integer string=w1896:string)  [unwired: 1 in]
                n908 = Number To Decimal String(number=w1899) -> (decimal integer string=w1898:string)  [unwired: 1 in]
                n909 = local read "Index"() -> (w1902:string)
                n910 = Strip Path(path=w1886) -> (stripped path=w1907:path)  [unwired: 1 out]
                n911 = call "Build Text2"("Temp"=w1863, "Index"=w1902, "Length"=w1896, "Width"=w1898) -> ("Result"=w1903:string)  [unwired: 10 in, 1 out]
                n912 = Replace Array Subset(array=w1893, new element=w1900, index (row)=13, index (col)=w1871) -> (w1895:string[][])
                n913 = Array Size(array=w1878) -> (size(s)=w1880:i32[])
                n914 = Path To String(path=w1907) -> (string=w1905:string)
                n915 = Number To Fractional String(number=w1908) -> (F-format string=w1887:string)  [unwired: 3 in]
                n916 = local read "New: Dielectric"() -> (w1909:dbl)
                n917 = Array Subset(array=w1878, index (row)=0, index (col)=0) -> (w1884:string[][])  [unwired: 2 in]
                n918 = Index Array(array=w1880, index=0) -> (element=w1879:i32)
                n919 = Replace Array Subset(array=w1895, new element=w1887, index (row)=15, index (col)=w1871) -> (w1894:string[][])
                n920 = Number To Fractional String(number=w1909) -> (F-format string=w1888:string)  [unwired: 3 in]
                n921 = Reshape Array(w1884, w1879) -> (w1872:string[])
                n922 = Concatenate Strings(w1905, "\\", w1903) -> (w1904:string)
                n923 = String To Path(string=w1904) -> (path=w1885:path)
                n924 = Search 1D Array(1D array=w1872, element=w1867) -> (index of element=w1876:i32)  [unwired: 1 in]
                n925 = Search 1D Array(1D array=w1872, element=w1866) -> (index of element=w1877:i32)  [unwired: 1 in]
                n926 = Equal?(x=w1876, y=w1873) -> (x = y?=w1874:bool)
                n927 = Equal?(x=w1877, y=w1873) -> (x = y?=w1875:bool)
                n928 = Replace Array Subset(array=w1894, new element=w1888, index (row)=7, index (col)=w1871) -> (w1870:string[][])
                n929 = case shown="False" w1874 {
                  tunnel: w1876 -> [_ _]
                  tunnel: w1870 -> [w1932 w1940]
                  tunnel: [w1931 w1939] -> w1869
                  tunnel: w1867 -> [_ w1938]
                  frame False {
                    n930 = local read "New: VT-Sat"() -> (w1934:dbl)
                    n931 = Number To Fractional String(number=w1934) -> (F-format string=w1930:string)  [unwired: 3 in]
                    n932 = Replace Array Subset(array=w1932, new element=w1930, index (row)=17, index (col)=1) -> (w1931:string[][])
                  }
                  frame True {
                    n933 = local read "New: VT-Sat"() -> (w1941:dbl)
                    n934 = Number To Fractional String(number=w1941) -> (F-format string=w1937:string)  [unwired: 3 in]
                    n935 = Build Array(w1938, w1937) -> (w1936:string[])
                    n936 = Insert Into Array(array=w1940, index (row)=17, new element=w1936) -> (w1939:string[][])  [unwired: 1 in]
                  }
                }
                n937 = case shown="False" w1875 {
                  tunnel: w1877 -> [_ _]
                  tunnel: w1869 -> [w1919 w1927]
                  tunnel: [w1918 w1926] -> w1868
                  tunnel: w1866 -> [_ w1924]
                  frame False {
                    n938 = local read "New: STS"() -> (w1921:dbl)
                    n939 = Number To Fractional String(number=w1921) -> (F-format string=w1917:string)  [unwired: 3 in]
                    n940 = Replace Array Subset(array=w1919, new element=w1917, index (row)=18, index (col)=1) -> (w1918:string[][])
                  }
                  frame True {
                    n941 = local read "New: STS"() -> (w1928:dbl)
                    n942 = Number To Fractional String(number=w1928) -> (F-format string=w1925:string)  [unwired: 3 in]
                    n943 = Build Array(w1924, w1925) -> (w1923:string[])
                    n944 = Insert Into Array(array=w1927, index (row)=18, new element=w1923) -> (w1926:string[][])  [unwired: 1 in]
                  }
                }
              }
              frame #1 {
                n945 = Equal?(x=w1945, y=w1944) -> (x = y?=w1943:bool)
                n946 = case shown="False" w1943 {
                  tunnel: w1945 -> [w1949 _]
                  tunnel: w1944 -> [w1948 _]
                  frame False {
                    n947 = Move(source path=w1949, 9:TRUE, 10:w1948) -> ()  [unwired: 2 in, 3 out]
                  }
                  frame True {
                  }
                }
              }
              frame #2 {
                n948 = local write "Data File"(w1951) -> ()
                n949 = call-poly <vilib>:"Write To Spreadsheet File.vi"("2D data"=w1950, "file path (dialog if empty)"=w1951) -> ()  [unwired: 6 in, 1 out]
              }
              frame #3 {
                w2009 = 0
                # "Moves to next file and displays new image/data"
                n950 = property on="Image Out" class="ImageControl"() -> (error out=w1971:errorcluster, "Image Center Position"=w1975:cluster{"X":u32, "Y":u32})  [unwired: 2 in, 1 out]
                n951 = local read "Data File"() -> (w2014:path)
                n952 = Strip Path(path=w2014) -> (stripped path=w2005:path, name=w2023:string)
                n953 = Unbundle(w1975) -> ("X"=w1973:u32)  [unwired: 1 out]
                n954 = local write "Data Folder"(w2005) -> ()
                n955 = Bundle("X"=w1973, 0) -> (w1974:cluster{"X":u32, i32})  [unwired: 1 in]
                n956 = property on="Image Out" class="ImageControl"(error in=w1971, "Image Center Position"=w1974) -> ()  [unwired: 1 in, 2 out]
                n957 = List Folder(path=w2005) -> (filenames=w2019:string[])  [unwired: 3 in, 3 out]
                n958 = Search 1D Array(1D array=w2019, element=w2023) -> (index of element=w2016:i32)  [unwired: 1 in]
                n959 = Array Size(array=w2019) -> (size(s)=w2015:i32)
                n960 = Decrement(x=w2015) -> (x-1=w2017:i32)
                n961 = Equal?(x=w2016, y=w2017) -> (x = y?=w2018:bool)
                n962 = local read "Folder Index"() -> (w1967:dbl)
                n963 = case shown="False" w2018 {
                  tunnel: w1967 -> [w2146 _]
                  tunnel: [w2145 0] -> w1966
                  frame False {
                    n964 = Increment(x=w2146) -> (x+1=w2145:dbl)
                  }
                  frame True {
                  }
                }
                n965 = invoke on="Image Out" class="ImageControl" method="Clear ROI"() -> ()  [unwired: 3 in, 3 out]
                n966 = local write "Folder Index"(w1966) -> ()
                n967 = Path To String(path=w2005) -> (string=w2024:string)
                n968 = Index Array(array=w2019, index=w1966) -> (element=w2020:string)
                n969 = local write "Data Name:"(w2020) -> ()
                n970 = Concatenate Strings(w2024, "\\", w2020) -> (w2022:string)
                n971 = String To Path(string=w2022) -> (path=w1965:path)
                n972 = local write "Data File"(w1965) -> ()
                n973 = local read "NumPts 2"() -> (w1956:dbl)
                n974 = local read "NumPts"() -> (w1957:dbl)
                n975 = call-poly <vilib>:"Read From Spreadsheet File.vi"("file path (dialog if empty)"=w1965) -> ("all rows"=w2011:string[][])  [unwired: 6 in, 4 out]
                n976 = call "Mobility-Vt Calculator-File.vi"("NumPts"=w1957, "Path"=w1965) -> ("XY Graph-Sat"=w1959:cluster{dbl[], dbl[]}[], "Output"=w1960:T8, "Index-Sat"=w1958:dbl)  [unwired: 5 in, 2 out]
                n977 = call "STS Calculator-File.vi"("NumPts"=w1956, "Path"=w1965) -> ("STS Index-Sat"=w1955:dbl, "XY Graph-Sat"=w1954:cluster{dbl[], dbl[]}[], "Ouput"=w1953:cluster{"STS-Sat":dbl, "STS-Lin":dbl})  [unwired: 5 in, 2 out]
                n978 = local write "MobVi Index"(w1958) -> ()
                n979 = local write "Slide"(w1958) -> ()
                n980 = local write "XY Graph"(w1959) -> ()
                n981 = local write "Index 2"(w1955) -> ()
                n982 = local write "XY Graph 2"(w1954) -> ()
                n983 = Unbundle By Name(w1960) -> ("Mobility-Sat"=w1964:dbl, "Vt-Sat"=w1963:dbl, "Mobility-Lin"=w1962:dbl, "Mobility-Lin"=w1961:dbl)
                n984 = Array Size(array=w2011) -> (size(s)=w2010:i32[])
                n985 = Unbundle By Name(w1953) -> ("STS-Sat"=w1952:dbl)
                n986 = local write "Calc: Mobility-Sat"(w1964) -> ()
                n987 = local write "Calc: Mobility-Lin"(w1961) -> ()
                n988 = local read "Image Folder"() -> (w1999:path)
                n989 = local write "Calc: VT-Sat"(w1963) -> ()
                n990 = local write "Calc: VT-Lin"(w1962) -> ()
                n991 = Decimate 1D Array(w1959) -> (w1994:cluster{dbl[], dbl[]}[])  [unwired: 1 out]
                n992 = Index Array(array=w2010, index=w2009) -> (element=w1990:i32)
                n993 = Decimate 1D Array(w1954) -> (w1984:cluster{dbl[], dbl[]}[])  [unwired: 1 out]
                n994 = Array Subset(array=w2011, index (row)=w2009, index (col)=w2009, length (col)=3) -> (w2012:string[][])  [unwired: 1 in]
                n995 = local write "Calc: STS"(w1952) -> ()
                n996 = List Folder(path=w1999) -> (filenames=w2004:string[])  [unwired: 3 in, 3 out]
                n997 = Array To Cluster(array=w1994) -> (cluster=w1996:T9)
                n998 = Array To Cluster(array=w1984) -> (cluster=w1982:T9)
                n999 = Reshape Array(w2012, w1990) -> (w1997:string[])
                n1000 = Subtract(x=w1990, y=20) -> (x-y=w1989:i32)
                n1001 = property on="Slide" class="Slide (strict)"("Scale.Maximum"=w1989) -> ()  [unwired: 2 in, 2 out]
                n1002 = Unbundle(w1996) -> ("[0]"=w1995:cluster{dbl[], dbl[]})  [unwired: 8 out]
                n1003 = Unbundle(w1982) -> ("[0]"=w1983:cluster{dbl[], dbl[]})  [unwired: 8 out]
                n1004 = Search 1D Array(1D array=w1997, element="Index:") -> (index of element=w2006:i32)  [unwired: 1 in]
                n1005 = Increment(x=w2006) -> (x+1=w2007:i32)
                n1006 = Unbundle(w1995) -> (w1986:dbl[], w1985:dbl[])
                n1007 = Unbundle(w1983) -> (w1981:dbl[], w1980:dbl[])
                n1008 = Array Subset(array=w1986, index=w1958, length=w1957) -> (w1993:dbl[])
                n1009 = Array Subset(array=w1985, index=w1958, length=w1957) -> (w1992:dbl[])
                n1010 = Array Subset(array=w1981, index=w1955, length=w1956) -> (w1988:dbl[])
                n1011 = Array Subset(array=w1980, index=w1955, length=w1956) -> (w1987:dbl[])
                n1012 = Index Array(array=w1997, index=w2007) -> (element=w2002:string)
                n1013 = local write "Array"(w1993) -> ()
                n1014 = local write "Index"(w2002) -> ()
                n1015 = local write "Array 2"(w1992) -> ()
                n1016 = local write "Array 8"(w1988) -> ()
                n1017 = local write "Array 7"(w1987) -> ()
                n1018 = while {
                  tunnel: w2004 -> [w2032]
                  tunnel: w2002 -> [w2030]
                  tunnel: [w2029] -> _
                  tunnel: [w2029] -> w2003
                  tunnel: w1990 -> [w2028]
                  i -> [w2029]
                  stop <- w2025 stop-if-true
                  n1019 = Index Array(array=w2032, index=w2029) -> (element=w2033:string)
                  n1020 = xnode "Match Regular Expression"("input string"=w2033, "regular expression"=w2030) -> ("whole match"=w2031:string)  [unwired: 4 in, 4 out]
                  n1021 = Equal?(x=w2031, y=w2030) -> (x = y?=w2027:bool)
                  n1022 = Equal?(x=w2028, y=w2029) -> (x = y?=w2026:bool)
                  n1023 = Or(x=w2027, y=w2026) -> (x .or. y?=w2025:bool)
                }
                n1024 = Path To String(path=w1999) -> (string=w2001:string)
                n1025 = Index Array(array=w2004, index=w2003) -> (element=w1978:string)
                n1026 = local write "Image Name"(w1978) -> ()
                n1027 = Empty String/Path?(string/path=w1978) -> (empty?=w1979:bool)
                n1028 = Concatenate Strings(w2001, "\\", w1978) -> (w2000:string)
                n1029 = String To Path(string=w2000) -> (path=w1977:path)
                n1030 = local read "No Image"() -> (w1976:path)
                n1031 = Select(t=w1976, s=w1979, f=w1977) -> (s? t:f=w1970:path)
                n1032 = local write "Image File"(w1970) -> ()
                n1033 = local read "Image Out"() -> (w1968:T2)
                n1034 = call "IMAQ ReadFile"("File Path"=w1970, "Image"=w1968) -> ("Image Out"=w1969:T2)  [unwired: 5 in, 4 out]
                n1035 = local write "Image Out"(w1969) -> ()
                n1036 = local write "Image Out 2"(w1969) -> ()
              }
              frame #4 {
                # "Output ROI data"
                n1037 = local read "Image Folder"() -> (w2148:path)
                n1038 = Build Path(base path=w2148, name or relative path="ROI") -> (appended path=w2150:path)
                n1039 = local read "Index"() -> (w2149:string)
                n1040 = Build Path(base path=w2150, name or relative path=w2149) -> (appended path=w2155:path)
                n1041 = invoke on="Image Out" class="ImageControl" method="Clear ROI"() -> (error out=w2154:errorcluster)  [unwired: 3 in, 2 out]
                n1042 = call <vilib>:"Check if File or Folder Exists.vi"("error in (no error)"=w2154, "path"=w2155) -> ("file or folder exists?"=w2152:bool, "dup path"=w2153:path)  [unwired: 7 in, 1 out]
                n1043 = case shown="True" w2152 {
                  tunnel: w2153 -> [_ w2156]
                  frame False {
                  }
                  frame True {
                    n1044 = Read from Text File(file (use dialog)=w2156) -> (text=w2160:string)  [unwired: 3 in, 3 out]
                    n1045 = property on="Image Out" class="ImageControl"() -> ("ROI"=w2157:T10)  [unwired: 2 in, 2 out]
                    n1046 = Unflatten From String(type=w2157, binary string=w2160) -> (value=w2158:T10, error out=w2159:errorcluster)  [unwired: 3 in, 1 out]
                    n1047 = property on="Image Out" class="ImageControl"(error in=w2159, "ROI"=w2158) -> ()  [unwired: 1 in, 2 out]
                  }
                }
              }
            }
            n1048 = flat-sequence {
              tunnel: [w1820] -> w1807
              tunnel: w1807 -> [w1834]
              frame #0 {
                # "Makes Empty File for Transformer Data"
                n1049 = local read "Data Folder"() -> (w1809:path)
                n1050 = Build Path(base path=w1809, name or relative path="Stats") -> (appended path=w1811:path)
                n1051 = call <vilib>:"Check if File or Folder Exists.vi"("path"=w1811) -> ("file or folder exists?"=w1812:bool, "dup path"=w1813:path)  [unwired: 8 in, 1 out]
                n1052 = case shown="False" w1812 {
                  tunnel: [w1817 w1819] -> w1814
                  tunnel: w1813 -> [w1818 w1819]
                  frame False {
                    n1053 = Create Folder(path (use dialog)=w1818) -> (created path=w1817:path)  [unwired: 2 in, 2 out]
                  }
                  frame True {
                  }
                }
                n1054 = Build Path(base path=w1814, name or relative path="Tranformer Data.txt") -> (appended path=w1816:path)
                n1055 = call-poly <vilib>:"Write To Spreadsheet File.vi"("append to file? (new file:F)"=TRUE, "file path (dialog if empty)"=w1816) -> ()  [unwired: 6 in, 1 out]
              }
              frame #1 {
                # "Adds Headers if they don't exist"
                n1056 = Concatenate Strings("Stats\\", "Tranformer Data.txt") -> (w1827:string)
                n1057 = local read "Data Folder"() -> (w1826:path)
                n1058 = Build Path(base path=w1826, name or relative path=w1827) -> (appended path=w1820:path)
                n1059 = call-poly <vilib>:"Read From Spreadsheet File.vi"("file path (dialog if empty)"=w1820) -> ("first row"=w1825:string[])  [unwired: 6 in, 4 out]
                n1060 = Search 1D Array(1D array=w1825, element="DeviceID") -> (index of element=w1823:i32)  [unwired: 1 in]
                n1061 = Equal?(x=w1823, y=0) -> (x = y?=w1821:bool)
                n1062 = case shown="False" w1821 {
                  tunnel: w1820 -> [w1831 _]
                  frame False {
                    n1063 = local read "Transformer \nHeaders"() -> (w1830:string[])
                    n1064 = call-poly <vilib>:"Write To Spreadsheet File.vi"("1D data"=w1830, "file path (dialog if empty)"=w1831) -> ()  [unwired: 6 in, 1 out]
                  }
                  frame True {
                  }
                }
              }
              frame #2 {
                # "Adds current device if it doesn't exist"
                n1065 = local read "Current \nRecord"() -> (w1837:string[])
                n1066 = Index Array(array=w1837, index=0) -> (element=w1836:string)
                n1067 = Concatenate Strings("Stats\\", "Tranformer Data.txt") -> (w1840:string)
                n1068 = local read "Data Folder"() -> (w1839:path)
                n1069 = local write "Current Device ID"(w1836) -> ()
                n1070 = local read "Current Device ID"() -> (w1846:string)
                n1071 = Build Path(base path=w1839, name or relative path=w1840) -> (appended path=w1838:path)
                n1072 = call-poly <vilib>:"Read From Spreadsheet File.vi"("file path (dialog if empty)"=w1838) -> ("all rows"=w1833:string[][])  [unwired: 6 in, 4 out]
                n1073 = Index Array(array=w1833, index (col)=0) -> (element=w1844:string[])  [unwired: 1 in]
                n1074 = Search 1D Array(1D array=w1844, element=w1846) -> (index of element=w1832:i32)  [unwired: 1 in]
                n1075 = Equal?(x=w1832, y=-1) -> (x = y?=w1835:bool)
                n1076 = case shown="False" w1835 {
                  tunnel: w1834 -> [w1848 w1861]
                  tunnel: w1832 -> [w1853 _]
                  tunnel: w1833 -> [w1854 _]
                  frame False {
                    n1077 = local read "Current \nRecord"() -> (w1852:string[])
                    n1078 = Replace Array Subset(array=w1854, new element=w1852, index (row)=w1853) -> (w1849:string[][])  [unwired: 1 in]
                    n1079 = flat-sequence {
                      tunnel: [w1855] -> _
                      tunnel: [w1856] -> _
                      tunnel: [w1856] -> w1851
                      tunnel: [w1855] -> w1850
                      tunnel: w1849 -> [w1856]
                      tunnel: w1848 -> [w1855]
                      tunnel: w1851 -> [w1858]
                      tunnel: w1850 -> [w1857]
                      frame #0 {
                        n1080 = Delete(path (use dialog)=w1855) -> ()  [unwired: 4 in, 3 out]
                      }
                      frame #1 {
                        n1081 = call-poly <vilib>:"Write To Spreadsheet File.vi"("append to file? (new file:F)"=TRUE, "2D data"=w1858, "file path (dialog if empty)"=w1857) -> ()  [unwired: 5 in, 1 out]
                      }
                    }
                  }
                  frame True {
                    n1082 = local read "Current \nRecord"() -> (w1860:string[])
                    n1083 = call-poly <vilib>:"Write To Spreadsheet File.vi"("append to file? (new file:F)"=TRUE, "1D data"=w1860, "file path (dialog if empty)"=w1861) -> ()  [unwired: 5 in, 1 out]
                  }
                }
              }
            }
          }
          event "Export": Mouse Down {
            n1084 = event-data() -> ()  [unwired: 1 in, 7 out]
            n1085 = call "OA_ConnectToOrigin.vi"() -> ("error out"=w2182:errorcluster, "Origin.IOApplication"=w2183:refnum<k7>)  [unwired: 8 in]
            n1086 = local read "Data Folder"() -> (w2161:path)
            n1087 = local read "Project"() -> (w2181:path)
            n1088 = call "OA_Load.vi"("error in (no error)"=w2182, "Path"=w2181, "Origin.IOApplication"=w2183) -> ("error out"=w2174:errorcluster, "Origin.IOApplication"=w2175:refnum<k7>)  [unwired: 1 out]
            n1089 = call "OAExecute.vi"("script"="document -m 3;", "Error IO"=w2174, "Origin.IOApplication"=w2175) -> ("Error IO Out"=w2172:errorcluster, "Origin.IOApplication"=w2173:refnum<k7>)  [unwired: 1 in, 1 out]
            n1090 = Build Path(base path=w2161, name or relative path="Stats") -> (appended path=w2162:path)
            n1091 = flat-sequence {
              tunnel: w2161 -> [w2203]
              tunnel: w2180 -> [w2202]
              tunnel: [w2192] -> w2185
              tunnel: [w2193] -> w2184
              tunnel: w2173 -> [w2197]
              tunnel: w2172 -> [w2196]
              tunnel: w2161 -> [w2219]
              tunnel: w2180 -> [w2218]
              tunnel: w2185 -> [w2214]
              tunnel: w2184 -> [w2215]
              tunnel: [w2209] -> w2179
              tunnel: [w2208] -> w2178
              tunnel: w2161 -> [w2230]
              tunnel: w2180 -> [w2229]
              tunnel: w2179 -> [w2225]
              tunnel: w2178 -> [w2224]
              tunnel: [w2223] -> w2177
              tunnel: [w2222] -> w2176
              tunnel: w2161 -> [w2245]
              tunnel: w2180 -> [w2244]
              tunnel: w2177 -> [w2239]
              tunnel: w2176 -> [w2238]
              tunnel: [w2236] -> w2170
              tunnel: [w2235] -> w2169
              frame #0 {
                n1092 = call "Param_Analysis.vi"("error in (no error)"=w2196, "Folder 2"=w2203, "Parameter String"="Mobility (cm^2/Vs):", "Parameter Name"="Mobility", "Folder"=w2202) -> ("error out"=w2199:errorcluster, "Array 4"=w2189:string[], "Array 3"=w2198:string[][])  [unwired: 3 in, 1 out]
                n1093 = call "Origin_Export.vi"("String 3"="[MobHistTab]Sheet1", "error in (no error)"=w2199, "Array"=w2198, "String 2"="[MOBvsLTable]Mobilities", "String"="pe_cd \"Mobility Chart\";", "Origin.IOApplication"=w2197, "Array 2"=w2189) -> ("reference out"=w2195:refnum<k7>, "error out"=w2194:errorcluster)  [unwired: 2 in, 1 out]
                n1094 = call "OAExecute.vi"("script"="window -a MOBvsLTable;\nwindow -s TV;", "Error IO"=w2194, "Origin.IOApplication"=w2195) -> ("Error IO Out"=w2192:errorcluster, "Origin.IOApplication"=w2193:refnum<k7>)  [unwired: 1 in, 1 out]
              }
              frame #1 {
                n1095 = call "Param_Analysis.vi"("error in (no error)"=w2214, "Folder 2"=w2219, "Parameter String"="On/Off Current:", "Parameter Name"="On_Off_Current", "Folder"=w2218) -> ("error out"=w2213:errorcluster, "Array 4"=w2207:string[], "Array 3"=w2210:string[][])  [unwired: 3 in, 1 out]
                n1096 = call "Origin_Export.vi"("String 3"="[OnOffHistTab]Sheet1", "error in (no error)"=w2213, "Array"=w2210, "String 2"="[OnOffTable]On/Off Ratios", "String"="pe_cd \"OnOff vs L\";", "Origin.IOApplication"=w2215, "Array 2"=w2207) -> ("reference out"=w2209:refnum<k7>, "error out"=w2208:errorcluster)  [unwired: 2 in, 1 out]
              }
              frame #2 {
                n1097 = call "Param_Analysis.vi"("Folder 2"=w2230, "Parameter String"="S.T.S. (V/decade):", "Parameter Name"="STS", "Folder"=w2229) -> ("Array 4"=w2221:string[], "Array 3"=w2226:string[][])  [unwired: 4 in, 2 out]
                n1098 = call "Origin_Export.vi"("String 3"="[SHistTab]Sheet1", "error in (no error)"=w2224, "Array"=w2226, "String 2"="[STable]Threshold Swing", "String"="pe_cd \"Threshold Swing vs L\";", "Origin.IOApplication"=w2225, "Array 2"=w2221) -> ("reference out"=w2222:refnum<k7>, "error out"=w2223:errorcluster)  [unwired: 2 in, 1 out]
              }
              frame #3 {
                n1099 = call "Param_Analysis.vi"("Folder 2"=w2245, "Parameter String"="Threshold V (V):", "Parameter Name"="Threshold_V", "Folder"=w2244) -> ("Array 4"=w2234:string[], "Array 3"=w2237:string[][])  [unwired: 4 in, 2 out]
                n1100 = call "Origin_Export.vi"("String 3"="[VtHistTab]Sheet1", "error in (no error)"=w2239, "Array"=w2237, "String 2"="[VtTable]Threshold Voltages", "String"="pe_cd \"Threshold Voltage vs L\";", "Origin.IOApplication"=w2238, "Array 2"=w2234) -> ("reference out"=w2236:refnum<k7>, "error out"=w2235:errorcluster)  [unwired: 2 in, 1 out]
              }
            }
            n1101 = call <vilib>:"Check if File or Folder Exists.vi"("path"=w2162) -> ("file or folder exists?"=w2187:bool, "dup path"=w2186:path)  [unwired: 8 in, 1 out]
            n1102 = case shown="False" w2187 {
              tunnel: w2186 -> [w2247 w2248]
              tunnel: [w2246 w2248] -> w2180
              frame False {
                n1103 = Create Folder(path (use dialog)=w2247) -> (created path=w2246:path)  [unwired: 2 in, 2 out]
              }
              frame True {
              }
            }
            n1104 = call "File Dialog"("start path"=w2162) -> ("selected path"=w2165:path)  [unwired: 11 in, 3 out]
            n1105 = Path To String(path=w2165) -> (string=w2164:string)
            n1106 = call "OAExecute.vi"("script"="pe_cd /;\npe_cd \"Mobility Chart\"; ", "Error IO"=w2169, "Origin.IOApplication"=w2170) -> ("Error IO Out"=w2166:errorcluster, "Origin.IOApplication"=w2167:refnum<k7>)  [unwired: 1 in, 1 out]
            n1107 = call "OASaveProject.vi"("path"=w2164, "Error IO"=w2166, "Origin.IOApplication"=w2167) -> ()  [unwired: 3 out]
          }
          event "Blank Button": Mouse Down {
            n1108 = event-data() -> ()  [unwired: 1 in, 7 out]
            n1109 = local read "Data File"() -> (w2256:path)
            n1110 = Strip Path(path=w2256) -> (stripped path=w2252:path, name=w2254:string)
            n1111 = Path To String(path=w2252) -> (string=w2251:string)
            n1112 = Concatenate Strings(w2251, "\\", "X_", w2254) -> (w2250:string)
            n1113 = String To Path(string=w2250) -> (path=w2249:path)
            n1114 = Move(source path=w2256, 10:w2249) -> ()  [unwired: 3 in, 3 out]
            n1115 = local write "Data File"(w2249) -> ()
          }
          event "Cancel Button": Mouse Down {
            (unwired) 6
            n1116 = event-data() -> ()  [unwired: 1 in, 7 out]
            n1117 = call "Simulate_Keyboard.vi"("Action"=2, "Virtual Key"=162) -> ()  [unwired: 7 in, 1 out]
          }
        }
        n1118 = Reciprocal(x=w485) -> (1/x=w484:sgl)
        n1119 = Multiply(x=w484, y=10) -> (x*y=w486:sgl)
        n1120 = case shown="\"EQUALS\"" w525 {
          tunnel: w499 -> [w574 w580 w584 w586 w590 w592 w594 w596 w598 w600 w602 w604 w606 w608 w610 w612 w614 w616 w618 w620 w622 w624 w626 w628 w630 w632 w634 w636 w638 w640 w642 w644 w646 w648 w650 w652 w654 w656 w658 w660 w662 w664 w666 w668 w670 w672 w674 w676 w678 w680 w682 w684 w686 w688 w690 w692 w694 w696 w698 w700 w702 w704 w706 w708 w710 w712 w714 w716 w718 w720 w722 w724 w726 w728 w730 w732 w734 w736 w738 w740 w742 w744 w746 w748 w750 w752 w754 w756 w758 w760 w762 w764 w766 w768 w770 w772 w774 w776 w778 w780 w782 w784 w786 w788 w790]
          tunnel: [w574 w579 w583 w586 w590 w592 w594 w596 w598 w600 w602 w604 w606 w608 w610 w612 w614 w616 w618 w620 w622 w624 w626 w628 w630 w632 w634 w636 w638 w640 w642 w644 w646 w648 w650 w652 w654 w656 w658 w660 w662 w664 w666 w668 w670 w672 w674 w676 w678 w680 w682 w684 w686 w688 w690 w692 w694 w696 w698 w700 w702 w704 w706 w708 w710 w712 w714 w716 w718 w720 w722 w724 w726 w728 w730 w732 w734 w736 w738 w740 w742 w744 w746 w748 w750 w752 w754 w756 w758 w760 w762 w764 w766 w768 w770 w772 w774 w776 w778 w780 w782 w784 w786 w788 w790] -> w524
          tunnel: w500 -> [w576 w578 w582 w588 w589 w591 w593 w595 w597 w599 w601 w603 w605 w607 w609 w611 w613 w615 w617 w619 w621 w623 w625 w627 w629 w631 w633 w635 w637 w639 w641 w643 w645 w647 w649 w651 w653 w655 w657 w659 w661 w663 w665 w667 w669 w671 w673 w675 w677 w679 w681 w683 w685 w687 w689 w691 w693 w695 w697 w699 w701 w703 w705 w707 w709 w711 w713 w715 w717 w719 w721 w723 w725 w727 w729 w731 w733 w735 w737 w739 w741 w743 w745 w747 w749 w751 w753 w755 w757 w759 w761 w763 w765 w767 w769 w771 w773 w775 w777 w779 w781 w783 w785 w787 w789]
          tunnel: [w575 w578 w582 w587 w589 w591 w593 w595 w597 w599 w601 w603 w605 w607 w609 w611 w613 w615 w617 w619 w621 w623 w625 w627 w629 w631 w633 w635 w637 w639 w641 w643 w645 w647 w649 w651 w653 w655 w657 w659 w661 w663 w665 w667 w669 w671 w673 w675 w677 w679 w681 w683 w685 w687 w689 w691 w693 w695 w697 w699 w701 w703 w705 w707 w709 w711 w713 w715 w717 w719 w721 w723 w725 w727 w729 w731 w733 w735 w737 w739 w741 w743 w745 w747 w749 w751 w753 w755 w757 w759 w761 w763 w765 w767 w769 w771 w773 w775 w777 w779 w781 w783 w785 w787 w789] -> w523
          tunnel: w486 -> [w573 w577 w581 w585 _ _ _ _ _ _ _ _ _ _ _ _ _ _ _ _ _ _ _ _ _ _ _ _ _ _ _ _ _ _ _ _ _ _ _ _ _ _ _ _ _ _ _ _ _ _ _ _ _ _ _ _ _ _ _ _ _ _ _ _ _ _ _ _ _ _ _ _ _ _ _ _ _ _ _ _ _ _ _ _ _ _ _ _ _ _ _ _ _ _ _ _ _ _ _ _ _ _ _ _ _]
          frame "DOWN" {
            n1121 = Add(x=w576, y=w573) -> (x+y=w575:sgl)
          }
          frame "LEFT" {
            n1122 = Subtract(x=w580, y=w577) -> (x-y=w579:sgl)
          }
          frame "RIGHT" {
            n1123 = Add(x=w584, y=w581) -> (x+y=w583:sgl)
          }
          frame "UP" {
            n1124 = Subtract(x=w588, y=w585) -> (x-y=w587:sgl)
          }
          frame "ENTER (num pad)" {
          }
          frame "' (quote)" {
          }
          frame "END" {
          }
          frame "EQUALS" {
          }
          frame "ESCAPE" {
          }
          frame "GRAVE (`)" {
          }
          frame "HOME" {
          }
          frame "INSERT" {
          }
          frame "LBRACKET" {
          }
          frame "LCONTROL" {
          }
          frame "L ALT" {
          }
          frame "LSHIFT" {
          }
          frame "LWIN" {
          }
          frame "MINUS" {
          }
          frame "MULTIPLY" {
          }
          frame "NEXT" {
          }
          frame "NUMLOCK" {
          }
          frame "NUMPAD_0" {
          }
          frame "NUMPAD_1" {
          }
          frame "NUMPAD_2" {
          }
          frame "NUMPAD_3" {
          }
          frame "NUMPAD_4" {
          }
          frame "NUMPAD_5" {
          }
          frame "NUMPAD_6" {
          }
          frame "NUMPAD_7" {
          }
          frame "NUMPAD_8" {
          }
          frame "NUMPAD_9" {
          }
          frame "PAUSE" {
          }
          frame "PERIOD" {
          }
          frame "PRIOR (PG UP)" {
          }
          frame "RBRACKET" {
          }
          frame "RCONTROL" {
          }
          frame "RETURN" {
          }
          frame "R ALT" {
          }
          frame "RSHIFT" {
          }
          frame "RWIN" {
          }
          frame "SCROLL" {
          }
          frame "SEMICOLON" {
          }
          frame "SLASH" {
          }
          frame "SPACE" {
          }
          frame "SUBTRACT" {
          }
          frame "TAB" {
          }
          frame "DIVIDE" {
          }
          frame "DELETE" {
          }
          frame "DECIMAL" {
          }
          frame "COMMA" {
          }
          frame "CAPITAL" {
          }
          frame "BACKSLASH" {
          }
          frame "BACK" {
          }
          frame "ADD" {
          }
          frame "F15" {
          }
          frame "F14" {
          }
          frame "F13" {
          }
          frame "F12" {
          }
          frame "F11" {
          }
          frame "F10" {
          }
          frame "F9" {
          }
          frame "F8" {
          }
          frame "F7" {
          }
          frame "F6" {
          }
          frame "F5" {
          }
          frame "F4" {
          }
          frame "F3" {
          }
          frame "F2" {
          }
          frame "F1" {
          }
          frame "Z" {
          }
          frame "Y" {
          }
          frame "X" {
          }
          frame "W" {
          }
          frame "V" {
          }
          frame "U" {
          }
          frame "T" {
          }
          frame "S" {
          }
          frame "R" {
          }
          frame "Q" {
          }
          frame "P" {
          }
          frame "O" {
          }
          frame "N" {
          }
          frame "M" {
          }
          frame "L" {
          }
          frame "K" {
          }
          frame "J" {
          }
          frame "I" {
          }
          frame "H" {
          }
          frame "G" {
          }
          frame "F" {
          }
          frame "E" {
          }
          frame "D" {
          }
          frame "C" {
          }
          frame "B" {
          }
          frame "A" {
          }
          frame "9" {
          }
          frame "8" {
          }
          frame "7" {
          }
          frame "6" {
          }
          frame "5" {
          }
          frame "4" {
          }
          frame "3" {
          }
          frame "2" {
          }
          frame "1" {
          }
          frame "0" {
          }
        }
        n1125 = Bundle(w502, w501, w516, w515, 0.0) -> (w514:cluster{dbl, dbl, dbl, dbl, dbl})  [unwired: 1 in]
        n1126 = Bundle("X"=w524, "Y"=w523) -> (w518:cluster{"X":sgl, "Y":sgl})  [unwired: 1 in]
        n1127 = Divide(x=20, y=w485) -> (x/y=w488:sgl)
        n1128 = property on="Image Out" class="ImageControl"("Image Center Position"=w518) -> ()  [unwired: 2 in, 2 out]
        n1129 = call "IMAQ Convert Rectangle to ROI (Polygon)"("Rectangle"=w514) -> ("ROI Descriptor"=w512:T3)  [unwired: 7 in, 2 out]
        n1130 = Bundle("Application Font", w488, w492, w492, w492, w492, w492, TRUE, w490) -> (w494:T16)  [unwired: 1 in]
        n1131 = property on="Image Out 2" class="ImageControl"("ROI"=w512) -> ()  [unwired: 2 in, 2 out]
        n1132 = Bundle(w490, w494, w490, w490) -> (w493:T17)  [unwired: 1 in]
        n1133 = property on="Image Out" class="ImageControl"() -> ("ROI"=w467:T10)  [unwired: 2 in, 2 out]
        n1134 = Unbundle By Name(w467) -> ("Contours"=w541:T13)
        n1135 = local read "Image Out"() -> (w496:T2)
        n1136 = call "IMAQ Clear Overlay"("Image"=w496) -> ("Image Out"=w495:T2)  [unwired: 9 in, 1 out]
        n1137 = Initialize Array(0) -> (w539:i32[])  [unwired: 1 in]
        n1138 = local read "Magnification"() -> (w530:u16)
        n1139 = Array Size(array=w541) -> (size(s)=w540:i32)
        n1140 = Build Array(0.505025, 0.252522, 0.127742, 0.050345, 0.031129) -> (w531:dbl[])
        n1141 = Array Subset(array=w531, index=w530, length=1) -> (w528:dbl[])
        n1142 = property on="Image Out" class="ImageControl"() -> ("ZoomInteger"=w520:cluster{"X":i32, "Y":i32})  [unwired: 2 in, 2 out]
        n1143 = To Double Precision Float(number=w528) -> (double precision float=w527:dbl[])
        n1144 = for {
          N: w540 -> [_]
          shift-right: [w813] -> _
          shift-left: w541 -> [w813]
          shift-right: [w811] -> w526
          shift-left: w539 -> [w810]
          tunnel: w527 -> [w809]
          shift-right: [w806] -> _
          shift-left: w495 -> [w808]
          tunnel: w493 -> [w801]
          i -> [w805]
          n1145 = Index Array(array=w813, index=w805) -> (element=w822:T18)
          n1146 = Unbundle(w822) -> ("Points"=w821:i32[])  [unwired: 2 out]
          n1147 = Array To Cluster(array=w821) -> (cluster=w820:T19)
          n1148 = Unbundle(w820) -> ("Points[0]"=w800:i32, "Points[1]"=w797:i32, "Points[2]"=w812:i32, "Points[3]"=w818:i32)  [unwired: 5 out]
          n1149 = Add(x=w800, y=10) -> (x+y=w798:i32)
          n1150 = Subtract(x=w797, y=w818) -> (x-y=w817:i32)
          n1151 = Subtract(x=w800, y=w812) -> (x-y=w819:i32)
          n1152 = Square(x=w817) -> (x^2=w815:i32)
          n1153 = Square(x=w819) -> (x^2=w816:i32)
          n1154 = Add(x=w816, y=w815) -> (x+y=w814:i32)
          n1155 = Square Root(x=w814) -> (sqrt(x)=w791:dbl)
          n1156 = Multiply(x=w791, y=0.5) -> (x*y=w794:dbl)
          n1157 = Add(x=w794, y=w797) -> (x+y=w796:dbl)
          n1158 = Bundle(w798, w796) -> (w807:cluster{i32, dbl})  [unwired: 1 in]
          n1159 = Multiply(x=w791, y=w809) -> (x*y=w804:dbl[])
          n1160 = Index Array(array=w804) -> (element=w803:dbl)  [unwired: 1 in]
          n1161 = Number To Fractional String(number=w803) -> (F-format string=w802:string)  [unwired: 3 in]
          n1162 = call "IMAQ Overlay Text"("BG Color (Transparent)"=u32 0, "Text Color (black)"=u32 16448250, "Font, Size & Style"=w801, "String"=w802, "Origin"=w807, "Image"=w808) -> ("Image Out"=w806:T2)  [unwired: 4 in, 1 out]
          n1163 = Build Array (concatenate)(w810, w804) -> (w811:dbl[])
          n1164 = local write "Numeric 3"(w791) -> ()
        }
        n1165 = local write "ROI Descriptor"(w467) -> ()
        n1166 = Unbundle(w520) -> ("X"=w519:i32)  [unwired: 1 out]
        n1167 = Add Array Elements(numeric array=w526) -> (sum=w537:dbl)
        n1168 = local write "Distances"(w526) -> ()
        n1169 = local write "Total Width"(w537) -> ()
        n1170 = local write "Zoom"(w519) -> ()
        n1171 = local read "Rec: Width"() -> (w468:dbl)
        n1172 = local read "Manual"() -> (w466:bool)
        n1173 = Not(x=w466) -> (.not. x?=w464:bool)
        n1174 = local read "Total Width"() -> (w470:dbl)
        n1175 = Equal To 0?(x=w470) -> (x = 0?=w465:bool)
        n1176 = And(x=w465, y=w464) -> (x .and. y?=w463:bool)
        n1177 = case shown="True" w463 {
          tunnel: w468 -> [_ w551]
          frame False {
          }
          frame True {
            n1178 = local write "New: Width"(w551) -> ()
          }
        }
        n1179 = Or(x=w465, y=w466) -> (x .or. y?=w469:bool)
        n1180 = case shown="False" w469 {
          tunnel: w470 -> [w552 _]
          frame False {
            n1181 = local write "New: Width"(w552) -> ()
          }
          frame True {
          }
        }
      }
    }
  }
  n1182 = Build Array("DeviceID", "Fabricator", "Deposition", "Date", "Sample", "Row", "Column", "L (um)", "W (um)", "Material", "Treatment", "TC (mM)", "Solvent", "C (%)", "ST (C)", "Drops", "Wait (s)", "RT (F)", "RH (%)", "Ramp (s)", "RPM", "Accel (RPM/s)", "Time (s)", "Mobility", "On/Off", "Vt", "S.T.S") -> (→"Transformer \nHeaders":string[])
